vi "main.vi"() -> ()   [LabVIEW 2021]
uses:
  TypeDef/InitCluster.ctl
  <vilib>/express/express shared/transition.llb/Dynamic To Waveform Array.vi
  <vilib>/express/express signal manip/GetorSetDDTAttributes/Set DDT Attributes/SetT0.vi
  <vilib>/express/express signal manip/GetorSetDDTAttributes/Set DDT Attributes/sub Set StartTimeStamp.vi
  <vilib>/express/express shared/transition.llb/Waveform Array To Dynamic.vi
  GlobalVar/GlobalRes.vi
  <vilib>/express/express signal manip/GetorSetDDTAttributes/Set DDT Attributes/Set DDT Properties.xnode
  <vilib>/express/express signal manip/GetorSetDDTAttributes/Set DDT Attributes/Set DDT Attributes.lvlib
panel:
  out "BufPulse":dbl
  out "Number of samples":i32
  out "Rate":dbl
  out "Ilość impulsów":dbl
  out "Czas impulsu":dbl
  out "Info":string
  in  "Stop Button":bool
  in  "Start Button":bool
  in  "Exit Button":bool
  in  "Tab Control":T1(tab)
  in  "Chart/Graph":bool
  in  "Ilosc_ai":u8=1 min=1 max=5
  in  "Offset":dbl=2.0 min=-2.0 max=2.0 step=0.1
  in  "Frequency":dbl=10.1
  in  "Amplitude":dbl=0.2 min=-0.2 max=0.2
  in  "Phase":dbl
  in  "Radio Buttons":T2(radio)
  in  "Test sygnału":bool
  in  "Offset SinZak":dbl=4.0 caption="Offset"
  in  "Funk_pom":enum32{"F:1", "F:2"}(radio)
  in  "fclkknob":dbl(knob) scale=0.0..3.0
  in  "fclk-zad":dbl=35.0 min=35.0 max=600.0
  in  "Uref":dbl=0.5 min=0.5 max=1.0
  out "SygZad Podg":dynamicdata(graph)
  in  "Num of samp":i32=1000
  in  "rate [Hz]":dbl=2000.0
  in  "rate [Hz] 2":dbl=2000.0
  in  "Num of samp 2":i32=1000
  out "T1+T2":dbl
  out "CE 2":dbl(graph)
  out "IN HI / IN LO":dynamicdata(graph)
  out "INT IN":dynamicdata(graph)
  out "INT OUT":dynamicdata(graph)
  out "GATE":dynamicdata(graph)
  out "COUNTER":dynamicdata(graph)
  out "IN HI/ IN LO":dynamicdata(graph)
  out "GATE":dynamicdata(graph)
  out "INT OUT":dynamicdata(graph)
  out "INT IN":dynamicdata(graph)
  out "COUNTER":dbl[](graph)
  # "Duration of\nopen gate"
  # "Number of impulses\nduring open gate"
  # "Rate and number of samples of \neach analog input channel"
  # "Double integration A/D converter test software"
  # "Institute of Automation - Department of Measurements and Control Systems"
  # "Step 1. Configure the input signal"
  # "In Alternating signal \"Offset\" means a peaks of sine wave.\nFor example, if \"Offset\" is set to 2,\nthen wave will be oscillate between -2 and 2.\nIn Noise signal, \"Offset means a value  \naround which the amplitude value oscillates."
  # "Test the signal"
  # "Step 2. Enter parameters of frequency and operating mode"
  # "Chose Chart\nor Graph"
  # "Number of\nanalog inputs"
  # "Noise signal"
  # "Constant signal"
  # "Alternating signal"
  # "Measurement\nfunctions of A/D"
  # "Frequency of\nA/D clock"
  # "If the pulse frequency is set to EXT\nor 35-600kHz, enter the set value in kHz here"
  # "Reference\nVoltage"
  # "Input signal preview"
  # "Number of Pulses per cycle"
  # "Real signal entering the converter"
  # "Integrator input"
  # "Integrator Output"
  # "Gate"
  # "Pulses"
  # "Integrator input"
  # "Integrator Output"
  # "Gate"
  # "Pulses"
  # "Real signal entering the converter"
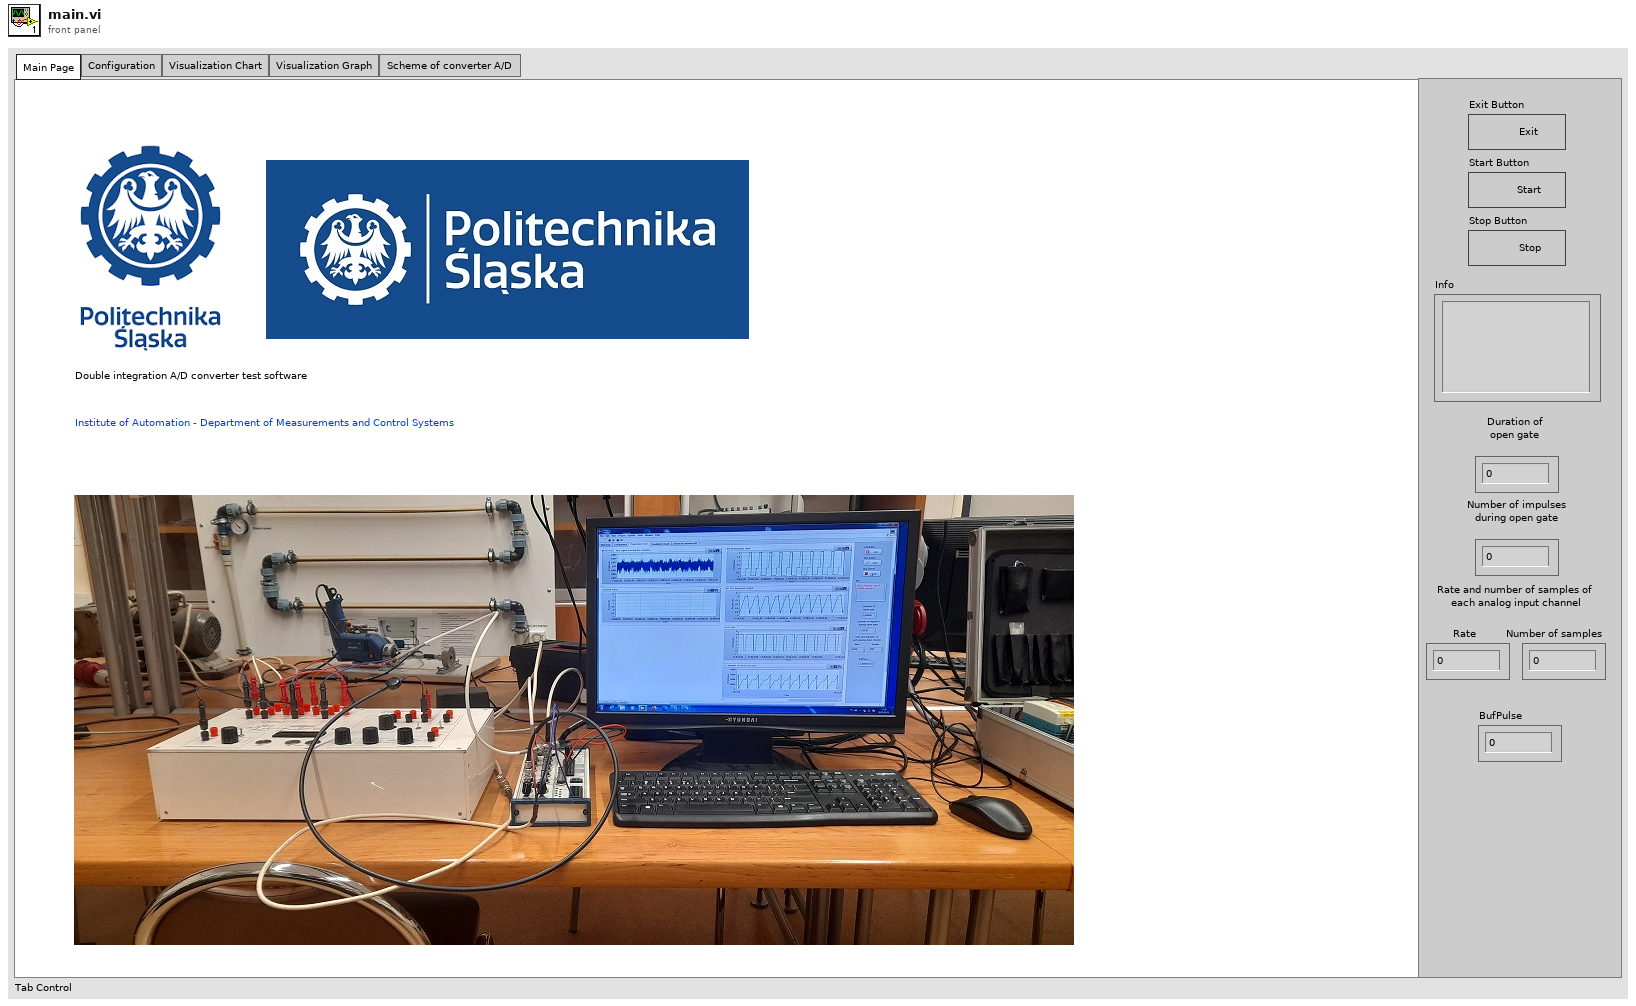
[diagram p1: front panel]
types:
  T1 = enum32{"Main Page", "Configuration", "Visualization Chart", "Visualization Graph", "Scheme of converter A/D "}
  T2 = enum32{"Sygnał przemienny", "Sygnał stały", "Sygnał zakłócony"}
  T3 = enum32{"Invalid", "Standard", "Closed", "Hidden", "Minimized", "Maximized"}
  T4 = enum32{"invalid app kind", "Development System", "Run Time System", "Student Edition", "Embedded LabVIEW", "Evaluation", "Custom"}
  T5 = enum8{"Enabled", "Disabled", "Disabled and Grayed Out"}
  T6 = typedef "InitCluster.ctl" = cluster{"Offset Ref":refnum<vi>, "Frequency Ref":refnum<vi>, "Amplitude Ref":refnum<vi>, "Phase Ref":refnum<vi>, "SygZad Podg Ref":refnum<vi>, "Test sygnału Ref":refnum<vi>, "Radio Buttons Ref":refnum<vi>, "Offset sin zakłócającej Ref":refnum<vi>, "fclkknob Ref":refnum<vi>, "fclk-zad Ref":refnum<vi>, "Info Ref":refnum<vi>}
  T7 = cluster{"Core":cluster{"Current VI Reference":refnum<vi>, "Close Panel on Exit?":bool}, "ClusterOUT":T6}
  T8 = cluster{"Current VI Reference":refnum<vi>, "Close Panel on Exit?":bool}
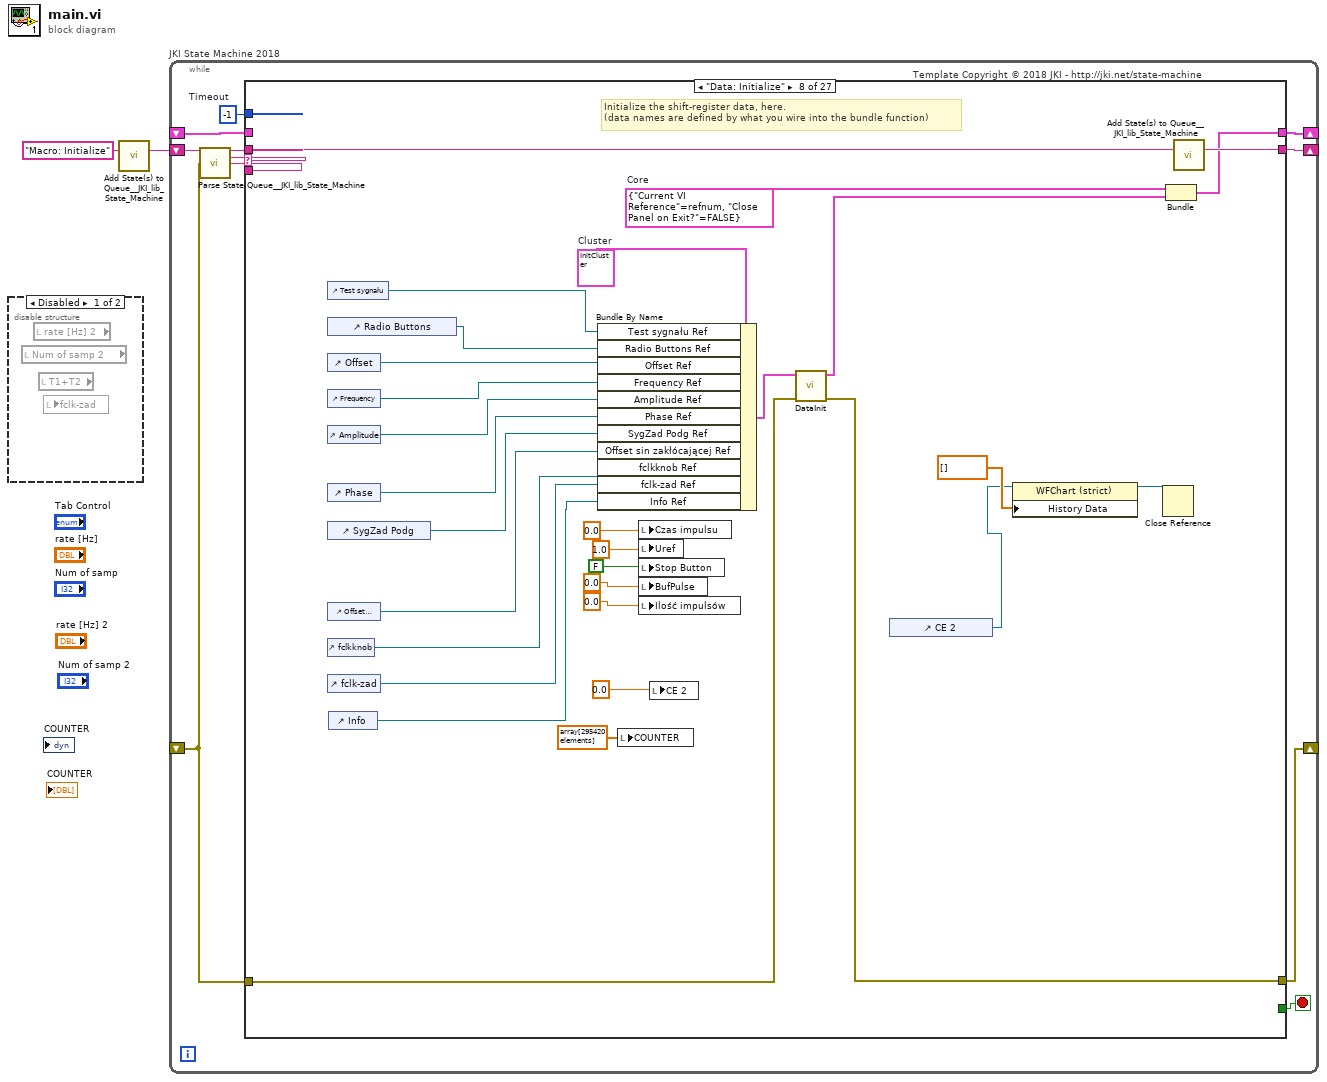
[diagram p0: block diagram]
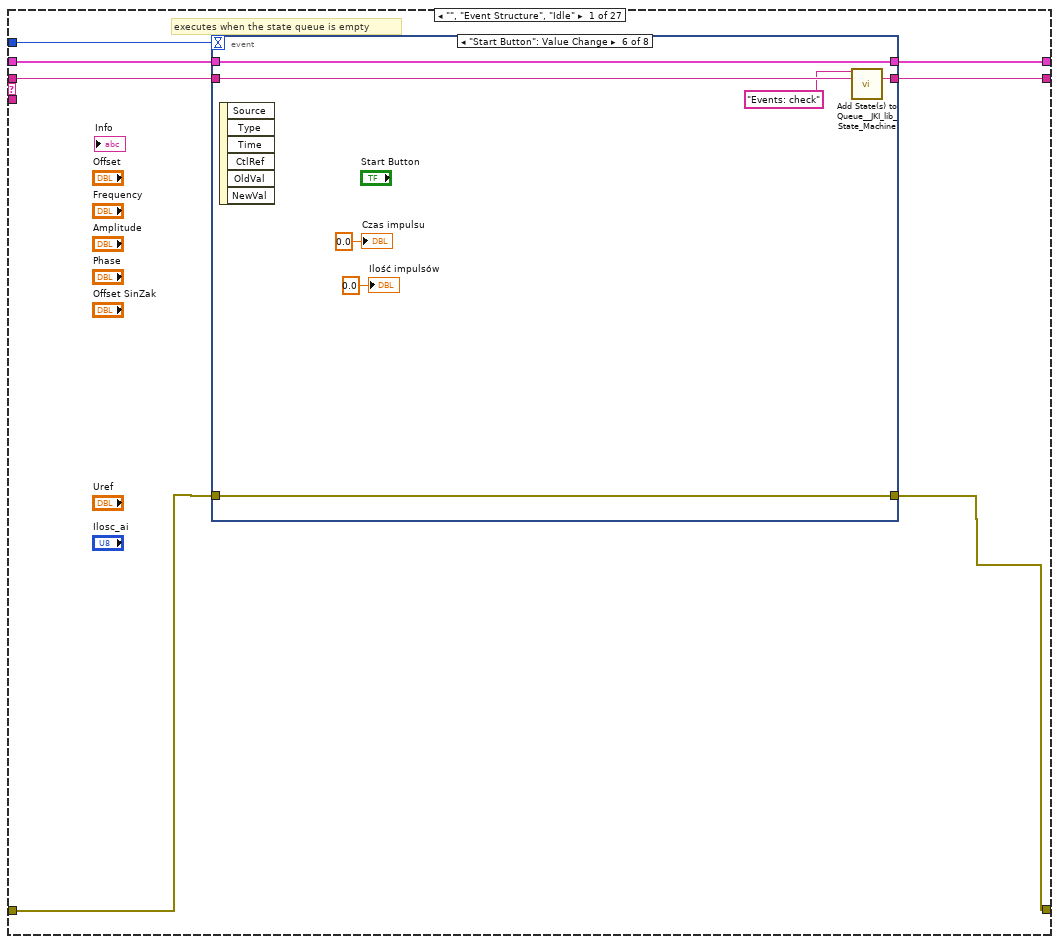
[diagram p3: hidden frame]
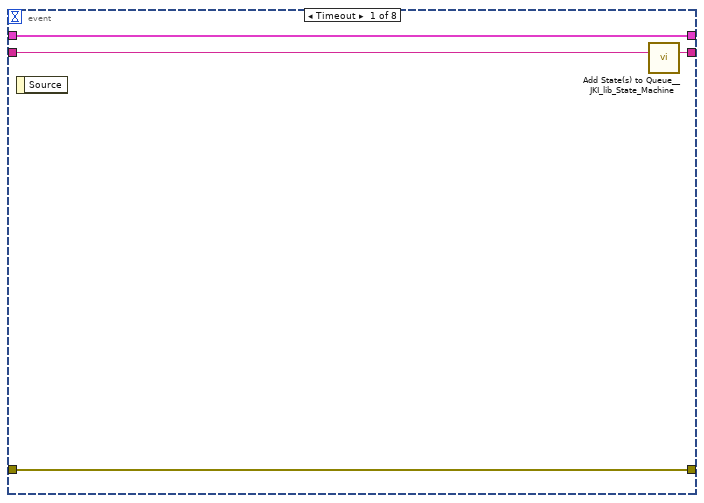
[diagram p4: hidden frame]
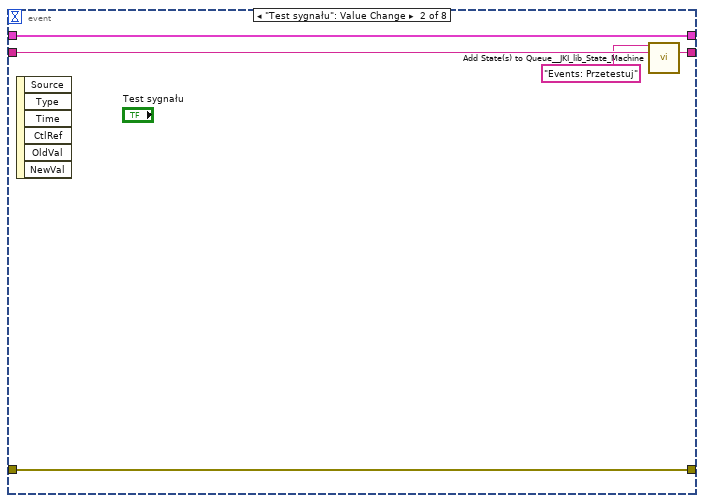
[diagram p5: hidden frame]
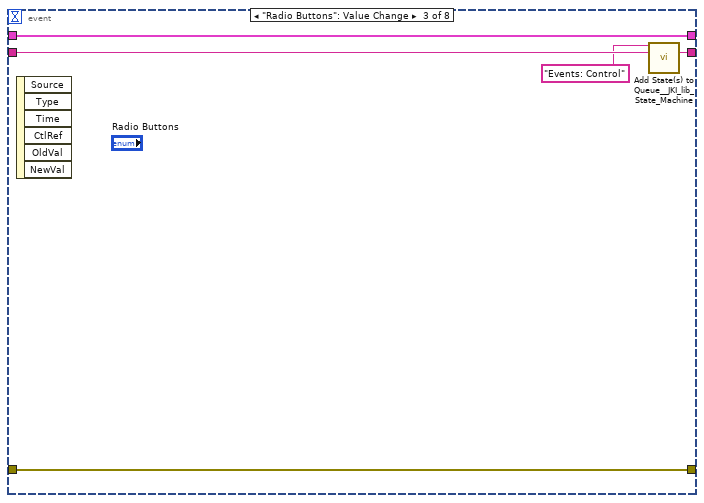
[diagram p6: hidden frame]
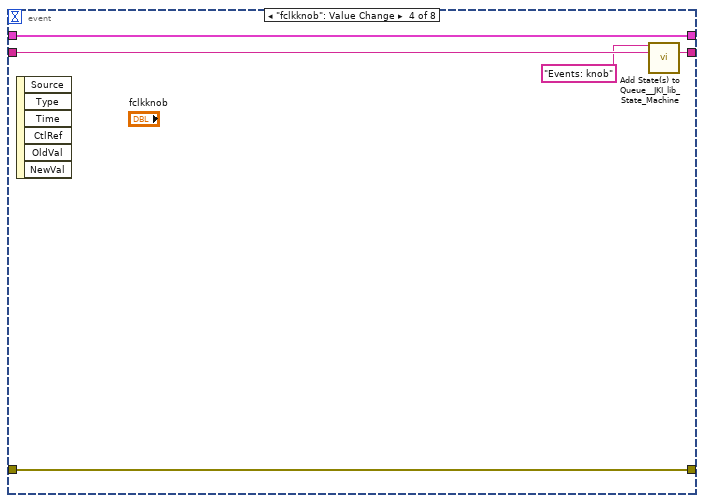
[diagram p7: hidden frame]
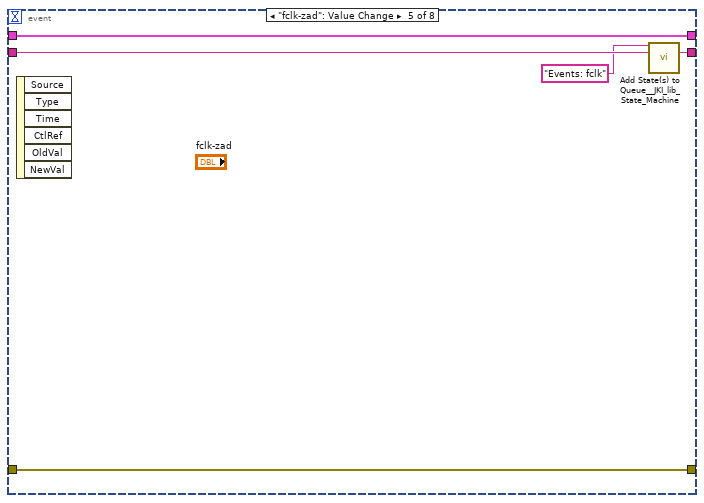
[diagram p8: hidden frame]
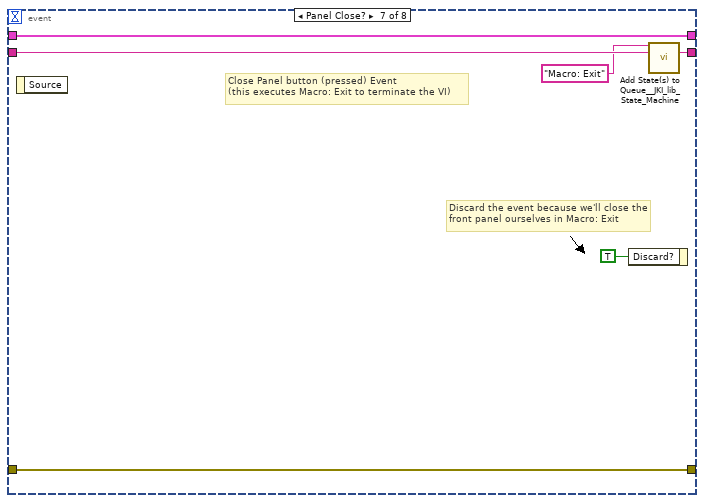
[diagram p9: hidden frame]
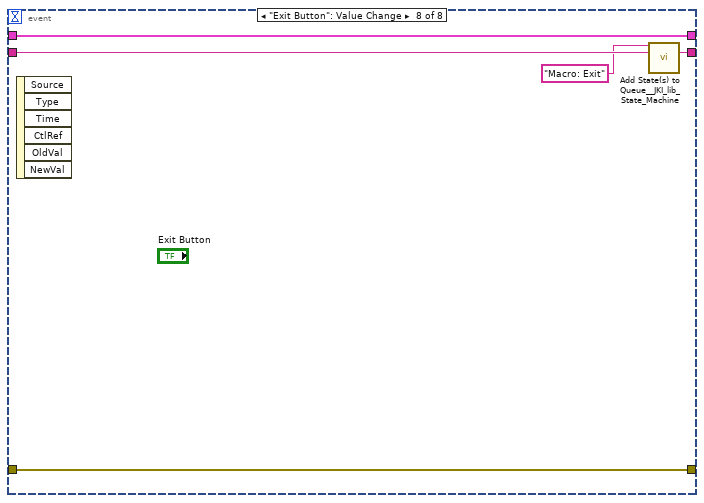
[diagram p10: hidden frame]
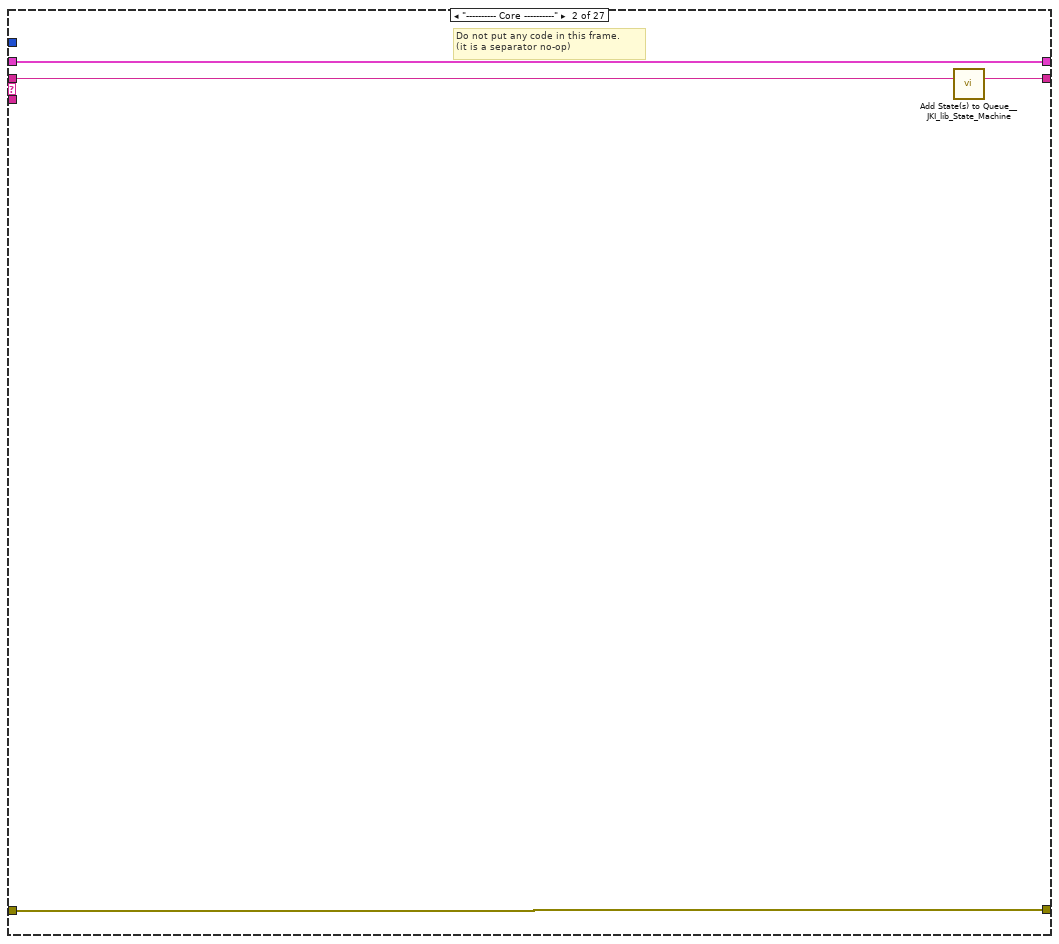
[diagram p11: hidden frame]
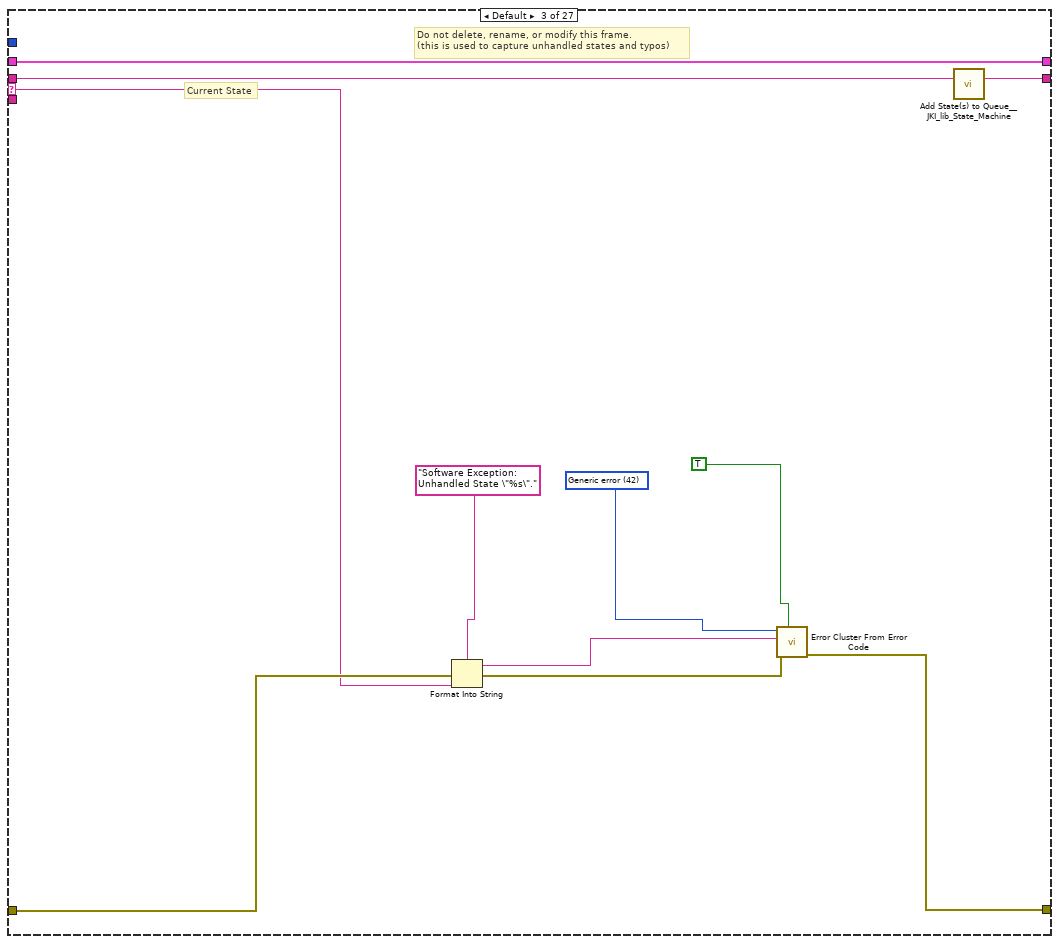
[diagram p12: hidden frame]
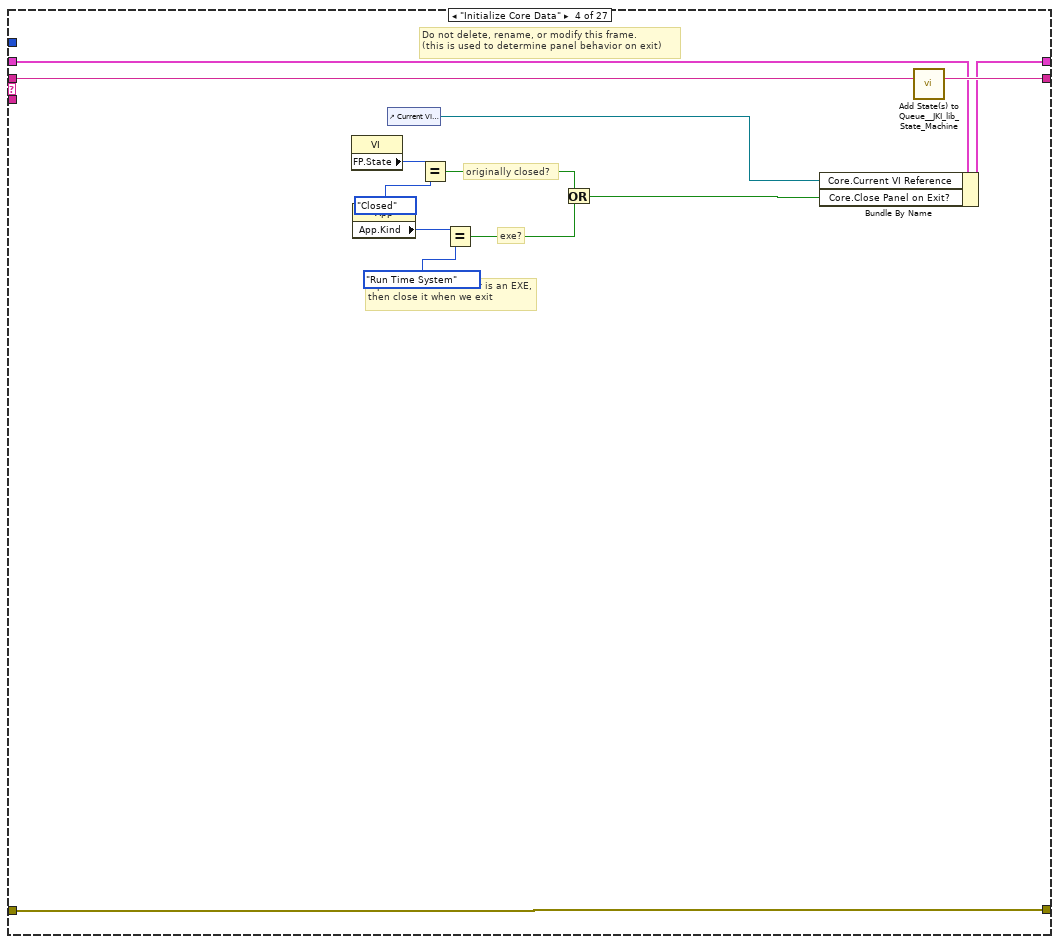
[diagram p13: hidden frame]
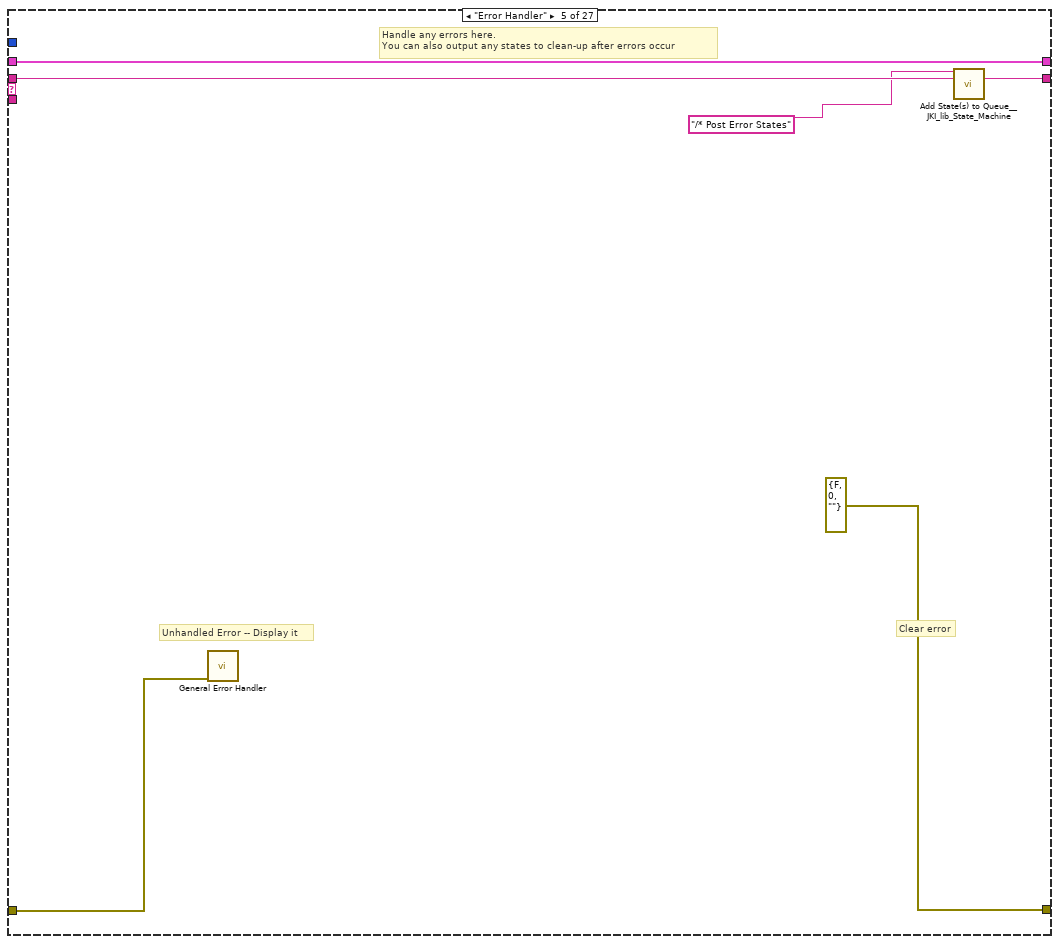
[diagram p14: hidden frame]
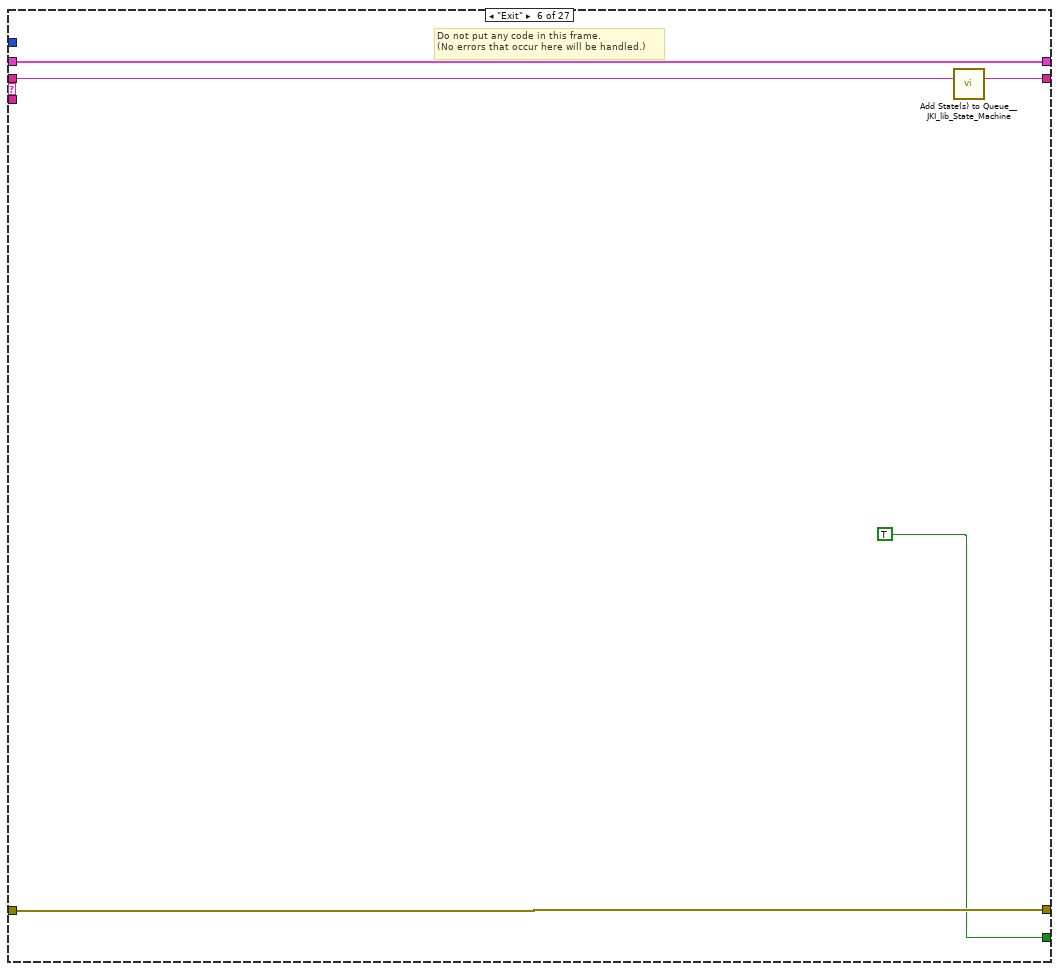
[diagram p15: hidden frame]
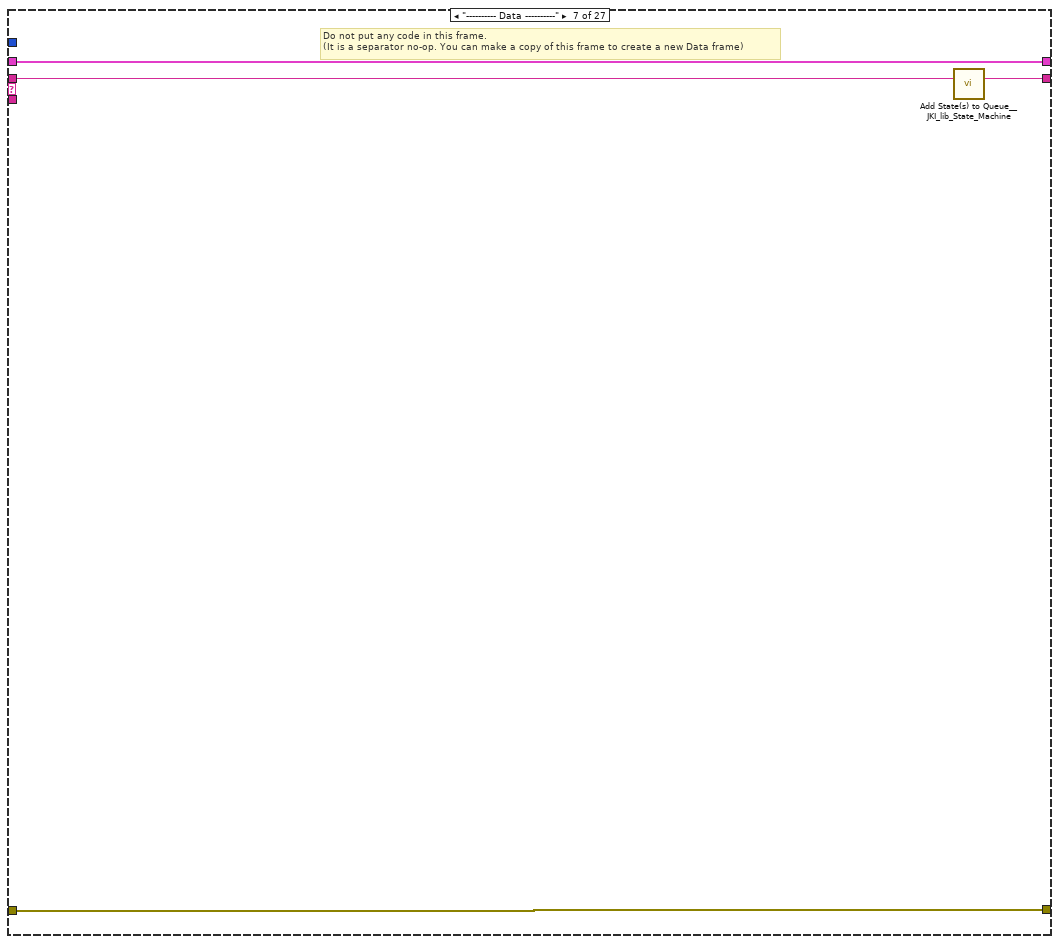
[diagram p16: hidden frame]
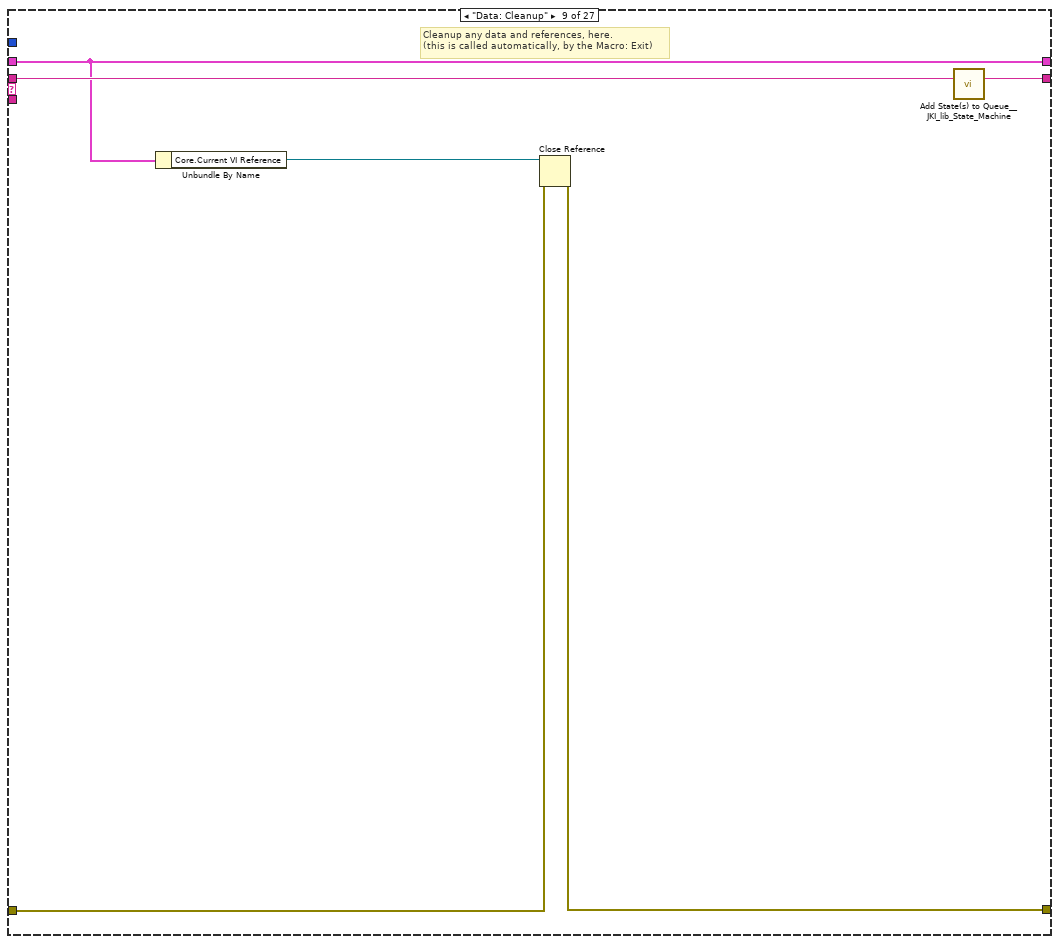
[diagram p17: hidden frame]
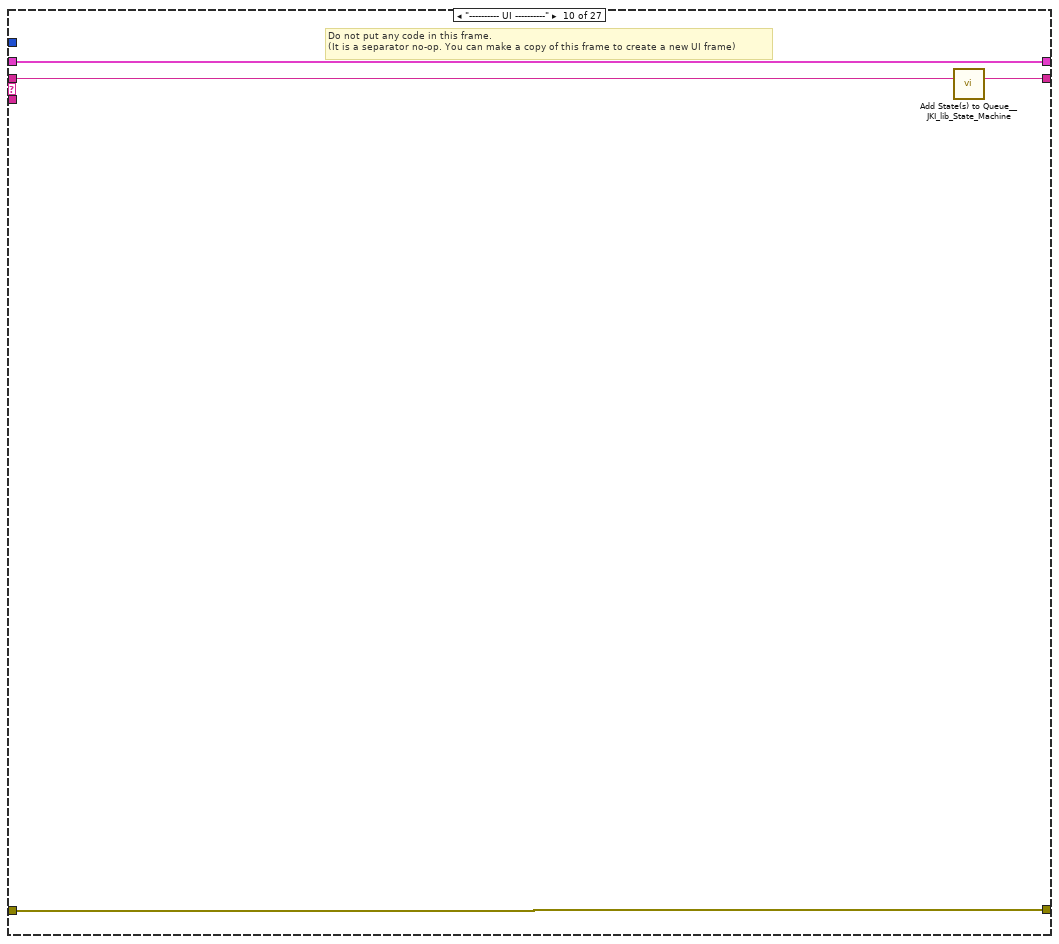
[diagram p18: hidden frame]
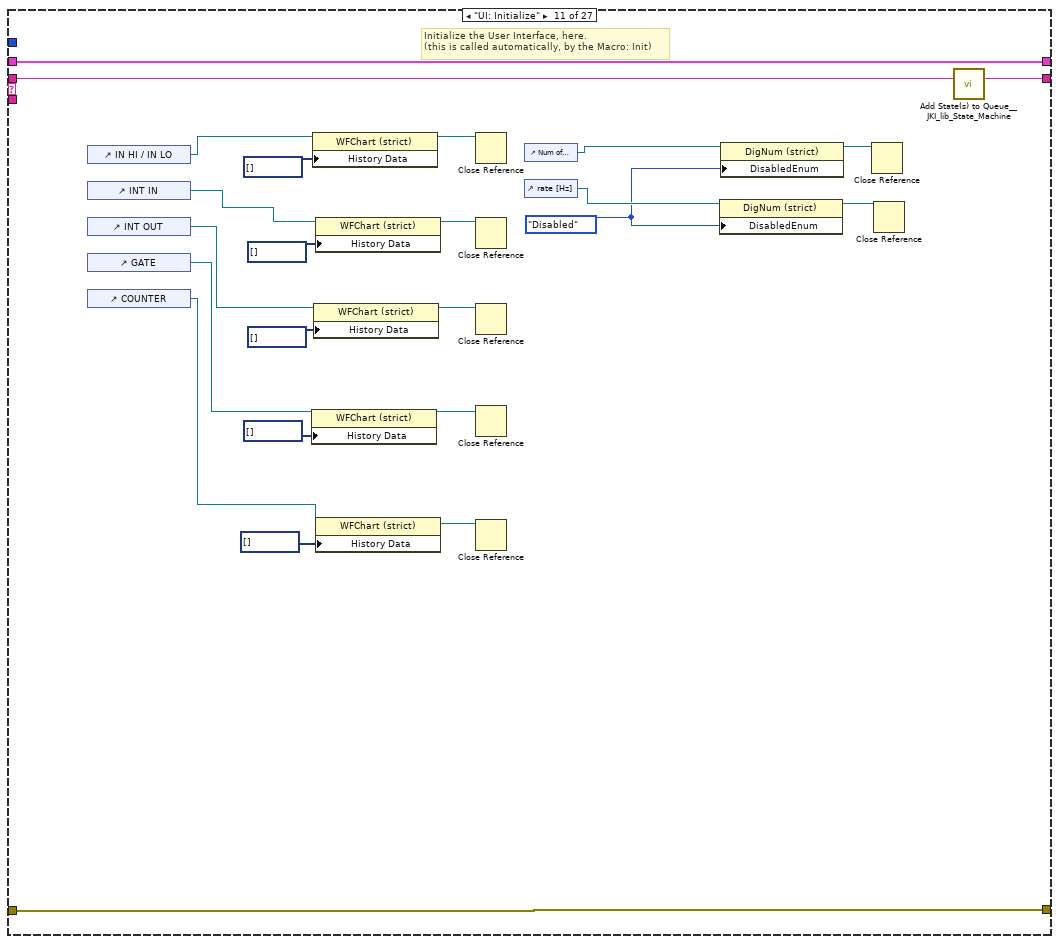
[diagram p19: hidden frame]
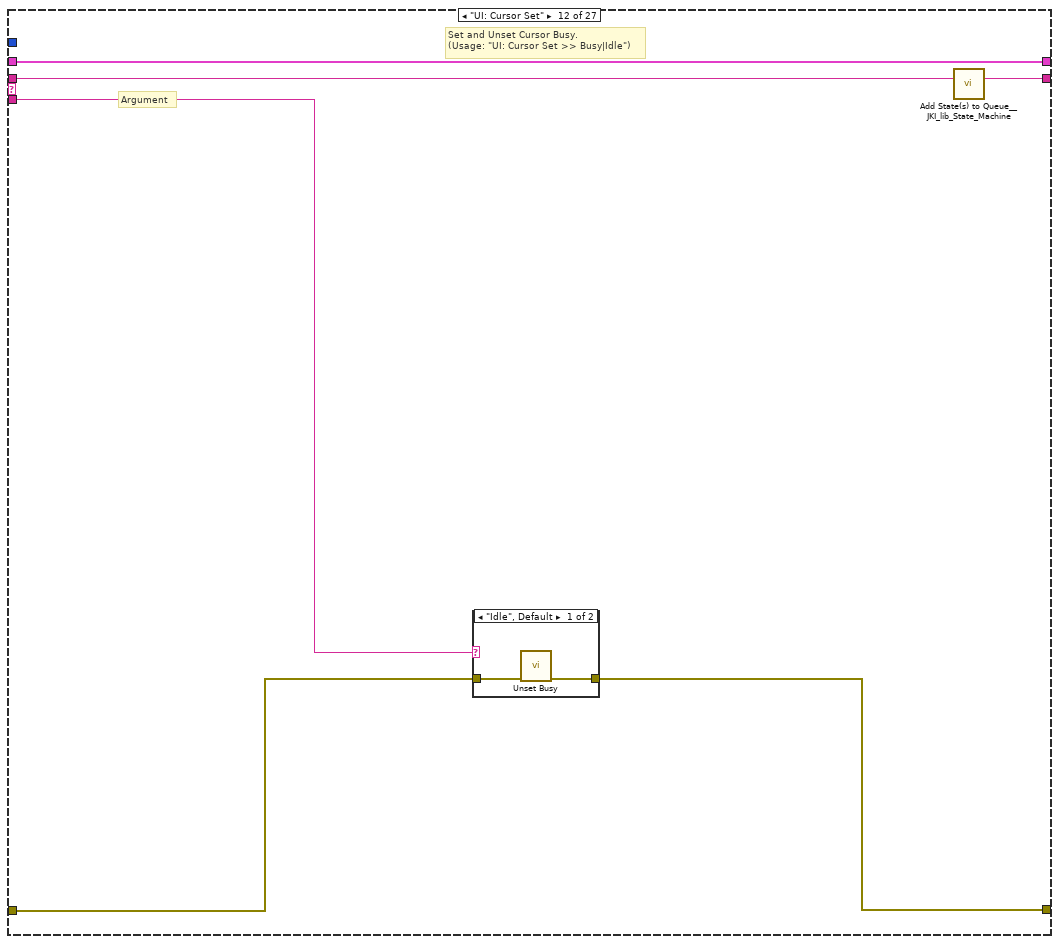
[diagram p20: hidden frame]
diagram:
  n1 = disable-structure shown="Disabled" {
    frame Disabled {
      n2 = local read "Num of samp 2"() -> ()  [unwired: 1 out]
      n3 = local read "rate [Hz] 2"() -> ()  [unwired: 1 out]
      n4 = local read "T1+T2"() -> ()  [unwired: 1 out]
      n5 = local read "fclk-zad"() -> ()  [unwired: 1 in]
    }
    frame Enabled {
    }
  }
  n6 = call <vilib>:"Add State(s) to Queue__JKI_lib_State_Machine.vi"("State(s) in (\"\")"="Macro: Initialize") -> ("States Out"=w2:string)  [unwired: 14 in]
  n7 = while "JKI State Machine 2018" {
    shift-right: [w7] -> _
    shift-left: _ -> [w6]
    shift-right: [w9] -> _
    shift-left: _ -> [w4]
    shift-right: [w8] -> _
    shift-left: w2 -> [w10]
    stop <- w3 stop-if-true
    w5 = -1  # Timeout
    # "Template Copyright © 2018 JKI - http://jki.net/state-machine"
    n8 = call <vilib>:"Parse State Queue__JKI_lib_State_Machine.vi"("State Queue"=w10, "Error In (no error)"=w4) -> ("Remaining States"=w12:string, "Current State"=w13:string, "Arguments"=w11:string)  [unwired: 11 in]
    n9 = case shown="\"Data: Initialize\"" w13 {
      selector: w13 -> [_ _ w67 _ _ _ _ _ _ _ _ _ _ _ _ _ _ _ _ _ _ _ _ _ _ _ _]
      tunnel: w12 -> [w20 w66 w71 w90 w96 w101 w105 w135 w141 w145 w169 w175 w186 w255 w260 w270 w274 w285 w337 w401 w441 w452 w551 w575 w639 w670 w700]
      tunnel: w11 -> [_ _ _ _ _ _ _ _ _ _ _ w170 w180 _ _ _ _ _ _ _ _ _ _ _ _ _ _]
      tunnel: w6 -> [w18 w63 w69 w83 w93 w99 w102 _ w136 w142 w167 w173 w182 w252 w257 w267 w271 w280 w334 w398 w439 w450 w549 w573 w636 w667 w698]
      tunnel: [w17 w64 w73 w87 errorcluster {"status"=FALSE, "code"=0, "source"=""} ("error out") w98 w103 w125 w137 w143 w166 w171 w183 w253 w258 w268 w272 w282 w332 w390 w436 w443 w518 w572 w624 w655 w686] -> w9
      tunnel: w4 -> [w16 w64 w72 w87 w92 w98 w103 w126 w138 w143 w166 w172 w184 w253 w258 w268 w272 w277 w333 w396 w438 w444 w546 w572 w624 w655 w685]
      tunnel: [w19 w65 w70 w89 w95 w100 w104 w134 w140 w144 w168 w174 w185 w254 w259 w269 w273 w284 w336 w400 w440 w451 w550 w574 w638 w669 w699] -> w8
      tunnel: [_ _ _ _ _ TRUE _ _ _ _ _ _ _ _ _ _ _ _ _ _ _ _ _ _ _ _ _] -> w3
      tunnel: [w15 w63 w69 w88 w93 w99 w102 w133 w136 w142 w167 w173 w182 w252 w257 w267 w271 w280 w334 w398 w439 w450 w549 w573 w636 w667 w698] -> w7
      tunnel: w5 -> [w14 _ _ _ _ _ _ _ _ _ _ _ _ _ _ _ _ _ _ _ _ _ _ _ _ _ _]
      frame "", "Event Structure", "Idle" {
        # "executes when the state queue is empty"
        n10 = event shown="[5] \"Start Button\": Value Change" {
          selector: _ -> [_ _ _ _ _ _ _ _]
          dyn-events: _ -> [_ _ _ _ _ _ _ _]
          timeout: w14 -> [_ _ _ _ _ _ _ _]
          tunnel: w20 -> [w24 w29 w34 w39 w44 w51 w57 w62]
          tunnel: [w23 w28 w33 w38 w43 w50 w56 w61] -> w19
          tunnel: w18 -> [w21 w26 w31 w36 w41 w48 w54 w59]
          tunnel: [w22 w27 w32 w37 w42 w49 w55 w60] -> w17
          tunnel: w16 -> [w22 w27 w32 w37 w42 w49 w55 w60]
          tunnel: [w21 w26 w31 w36 w41 w48 w54 w59] -> w15
          event Timeout {
            n11 = event-data() -> ()  [unwired: 1 in, 1 out]
            n12 = call <vilib>:"Add State(s) to Queue__JKI_lib_State_Machine.vi"("State(s) in (\"\")"=w24) -> ("States Out"=w23:string)  [unwired: 14 in]
          }
          event "Test sygnału": Value Change {
            n13 = event-data() -> ()  [unwired: 1 in, 6 out]
            n14 = call <vilib>:"Add State(s) to Queue__JKI_lib_State_Machine.vi"("State(s) in Front (\"\")"="Events: Przetestuj", "State(s) in (\"\")"=w29) -> ("States Out"=w28:string)  [unwired: 13 in]
          }
          event "Radio Buttons": Value Change {
            n15 = event-data() -> ()  [unwired: 1 in, 6 out]
            n16 = call <vilib>:"Add State(s) to Queue__JKI_lib_State_Machine.vi"("State(s) in Front (\"\")"="Events: Control", "State(s) in (\"\")"=w34) -> ("States Out"=w33:string)  [unwired: 13 in]
          }
          event "fclkknob": Value Change {
            n17 = event-data() -> ()  [unwired: 1 in, 6 out]
            n18 = call <vilib>:"Add State(s) to Queue__JKI_lib_State_Machine.vi"("State(s) in Front (\"\")"="Events: knob", "State(s) in (\"\")"=w39) -> ("States Out"=w38:string)  [unwired: 13 in]
          }
          event "fclk-zad": Value Change {
            n19 = event-data() -> ()  [unwired: 1 in, 6 out]
            n20 = call <vilib>:"Add State(s) to Queue__JKI_lib_State_Machine.vi"("State(s) in Front (\"\")"="Events: fclk", "State(s) in (\"\")"=w44) -> ("States Out"=w43:string)  [unwired: 13 in]
          }
          event "Start Button": Value Change {
            n21 = event-data() -> ()  [unwired: 1 in, 6 out]
            n22 = call <vilib>:"Add State(s) to Queue__JKI_lib_State_Machine.vi"("State(s) in Front (\"\")"="Events: check", "State(s) in (\"\")"=w51) -> ("States Out"=w50:string)  [unwired: 13 in]
            "Czas impulsu" <- 0.0 ("Czas impulsu")
            "Ilość impulsów" <- 0.0 ("Ilość impulsów")
          }
          event Panel Close? {
            # "Discard the event because we'll close the front panel ourselves in Macro: Exit"
            # "Close Panel button (pressed) Event\n(this executes Macro: Exit to terminate the VI)"
            n23 = event-data() -> ()  [unwired: 1 in, 1 out]
            n24 = event-data("Discard?"=TRUE) -> ()  [unwired: 1 in, 1 out]
            n25 = call <vilib>:"Add State(s) to Queue__JKI_lib_State_Machine.vi"("State(s) in Front (\"\")"="Macro: Exit", "State(s) in (\"\")"=w57) -> ("States Out"=w56:string)  [unwired: 13 in]
          }
          event "Exit Button": Value Change {
            n26 = event-data() -> ()  [unwired: 1 in, 6 out]
            n27 = call <vilib>:"Add State(s) to Queue__JKI_lib_State_Machine.vi"("State(s) in Front (\"\")"="Macro: Exit", "State(s) in (\"\")"=w62) -> ("States Out"=w61:string)  [unwired: 13 in]
          }
        }
      }
      frame "---------- Core ----------" {
        # "Do not put any code in this frame.\n(it is a separator no-op)"
        n28 = call <vilib>:"Add State(s) to Queue__JKI_lib_State_Machine.vi"("State(s) in (\"\")"=w66) -> ("States Out"=w65:string)  [unwired: 14 in]
      }
      frame Default {
        w76 = 42 items=["No error", "Argument error", "Memory is full", "Out of zone", "End of file", "File already open", "Generic file I/O error", "File not found", "File permission error", "Disk is full", "Duplicate path", "Too many files open", "System feature not enabled", "Resource file not found", "Cannot add resource", "Resource not found", "Image not found", "Image memory error", "Pen does not exist", "Config type invalid", "Config token not found", "Config parse error", "Config memory error", "Bad external code format", "Bad external code offset", "External code not present", "Null window", "Destroy window error", "Null menu", "Print aborted", "Bad print record", "Print driver error", "Windows error during printing", "Memory error during printing", "Print dialog error", "Generic print error", "Invalid device refnum", "Device not found", "Device parameter error", "Device unit error", "Cannot open device", "Device call aborted", "Generic error", "Cancelled by user", "Object ID too low", "Object ID too high", "Object not in heap", "Unknown heap", "Unknown object (invalid DefProc)", "Unknown object (DefProc not in table)", "Message out of range", "Invalid (null) method", "Unknown message", "Manager call not supported", "Bad address", "Network operation in progress", "Network operation timed out", "Connection is busy", "Network attribute not supported", "Network error", "Address in use", "System out of memory", "Connection aborted", "Connection refused", "Not connected", "Already connected", "Connection closed", "Initialization error (interapplication manager)", "Bad occurrence", "Wait on unbound occurrence handler", "Occurrence queue overflow", "Datalog type conflict", "Unused", "Unrecognized type (interapplication manager)", "Memory corrupt", "Failed to make temporary DLL", "Old CIN version", "Drag socket not found", "Failed to load drop-object", "Failed to register OLE object", "Failed to release OLE object", "Format specifier type mismatch", "Unknown format specifier", "Too few format specifiers", "Too many format specifiers", "Scan failed", "Newer CIN version", "Error converting to variant", "Runtime menu error", "Password tampered", "Variant attribute not found", "Incompatible variant data type", "Event data is not available", "Event Store is not present", "Occurrence is not found", "Event Queue is not created", "Event info is not available", "Refnum passed is NULL", "Error retrieving Class GUID", "Error retrieving CoClass GUID", "Error retrieving TypeLib GUID.", "Bad built application magic bytes.", "Specific driver is different from the specific driver associated with the Logical Name.", "There is no session opened to the class driver.", "Max Error", "MAX - Error with config objects", "MAX - Error loading configuration", "MAX - Group not supported"]
        # "Current State"
        # "Do not delete, rename, or modify this frame.\n(this is used to capture unhandled states and typos)"
        n29 = Format Into String(format string="Software Exception: Unhandled State \"%s\"." ("message"), error in=w72, w67) -> (resulting string=w75:string, error out=w74:errorcluster)  [unwired: 1 in]
        n30 = call <vilib>:"Error Cluster From Error Code.vi"("show call chain? (False)"=TRUE, "error in (no error)"=w74, "error message (\"\")"=w75, "error code (0)"=w76) -> ("error out"=w73:errorcluster)  [unwired: 5 in]
        n31 = call <vilib>:"Add State(s) to Queue__JKI_lib_State_Machine.vi"("State(s) in (\"\")"=w71) -> ("States Out"=w70:string)  [unwired: 14 in]
      }
      frame "Initialize Core Data" {
        # "Do not delete, rename, or modify this frame.\n(this is used to determine panel behavior on exit)"
        # "originally closed?"
        # "exe?"
        # "If panel starts closed or is an EXE, then close it when we exit"
        n32 = property class="VI"() -> ("FP.State"=w80:T3)  [unwired: 2 in, 2 out]
        n33 = property class="App"() -> ("App.Kind"=w86:T4)  [unwired: 2 in, 2 out]
        n34 = control-ref of="Current VI Reference"() -> (w81:refnum<vi>)
        n35 = Equal?(x=w80, y=T3."Closed" ("Front Panel Window:State")) -> (x = y?=w78:bool)
        n36 = Equal?(x=w86, y=T4."Run Time System" ("Application:Kind")) -> (x = y?=w84:bool)
        n37 = Or(x=w78, y=w84) -> (x .or. y?=w82:bool)
        n38 = Bundle By Name(cluster=w83, "Core.Current VI Reference"=w81, "Core.Close Panel on Exit?"=w82) -> (w88:T7)
        n39 = call <vilib>:"Add State(s) to Queue__JKI_lib_State_Machine.vi"("State(s) in (\"\")"=w90) -> ("States Out"=w89:string)  [unwired: 14 in]
      }
      frame "Error Handler" {
        # "Unhandled Error -- Display it"
        # "Handle any errors here.\nYou can also output any states to clean-up after errors occur"
        # "Clear error"
        n40 = call <vilib>:"General Error Handler.vi"("error in (no error)"=w92) -> ()  [unwired: 10 in, 5 out]
        n41 = call <vilib>:"Add State(s) to Queue__JKI_lib_State_Machine.vi"("State(s) in Front (\"\")"="/* Post Error States", "State(s) in (\"\")"=w96) -> ("States Out"=w95:string)  [unwired: 13 in]
      }
      frame "Exit" {
        # "Do not put any code in this frame.\n(No errors that occur here will be handled.)"
        n42 = call <vilib>:"Add State(s) to Queue__JKI_lib_State_Machine.vi"("State(s) in (\"\")"=w101) -> ("States Out"=w100:string)  [unwired: 14 in]
      }
      frame "---------- Data ----------" {
        # "Do not put any code in this frame.\n(It is a separator no-op. You can make a copy of this frame to create a new Data frame)"
        n43 = call <vilib>:"Add State(s) to Queue__JKI_lib_State_Machine.vi"("State(s) in (\"\")"=w105) -> ("States Out"=w104:string)  [unwired: 14 in]
      }
      frame "Data: Initialize" {
        w131 = T6 {"Offset Ref"=refnum, "Frequency Ref"=refnum, "Amplitude Ref"=refnum, "Phase Ref"=refnum, "SygZad Podg Ref"=refnum, "Test sygnału Ref"=refnum, "Radio Buttons Ref"=refnum, "Offset sin zakłócającej Ref"=refnum, "fclkknob Ref"=refnum, "fclk-zad Ref"=refnum, "Info Ref"=refnum}  # Cluster
        w132 = T8 {"Current VI Reference"=refnum, "Close Panel on Exit?"=FALSE}  # Core
        # "Initialize the shift-register data, here.\n(data names are defined by what you wire into the bundle function)"
        n44 = control-ref of="Test sygnału"() -> (w121:refnum<vi>)
        n45 = control-ref of="Radio Buttons"() -> (w120:refnum<vi>)
        n46 = control-ref of="Offset"() -> (w130:refnum<vi>)
        n47 = control-ref of="Frequency"() -> (w129:refnum<vi>)
        n48 = control-ref of="Amplitude"() -> (w128:refnum<vi>)
        n49 = control-ref of="Phase"() -> (w127:refnum<vi>)
        n50 = control-ref of="SygZad Podg"() -> (w122:refnum<vi>)
        n51 = control-ref of="Offset SinZak"() -> (w119:refnum<vi>)
        n52 = control-ref of="fclkknob"() -> (w118:refnum<vi>)
        n53 = control-ref of="fclk-zad"() -> (w117:refnum<vi>)
        n54 = control-ref of="Info"() -> (w116:refnum<vi>)
        n55 = Bundle By Name(cluster=w131, "Test sygnału Ref"=w121, "Radio Buttons Ref"=w120, "Offset Ref"=w130, "Frequency Ref"=w129, "Amplitude Ref"=w128, "Phase Ref"=w127, "SygZad Podg Ref"=w122, "Offset sin zakłócającej Ref"=w119, "fclkknob Ref"=w118, "fclk-zad Ref"=w117, "Info Ref"=w116) -> (w124:T6)
        n56 = local write "COUNTER"(dbl[] array[295420 elements] ("COUNTER")) -> ()
        n57 = local write "Czas impulsu"(0.0 ("Czas impulsu")) -> ()
        n58 = local write "Uref"(1.0 ("Uref")) -> ()
        n59 = local write "Stop Button"(FALSE ("Stop Button")) -> ()
        n60 = local write "BufPulse"(0.0 ("Numeric")) -> ()
        n61 = local write "Ilość impulsów"(0.0 ("Ilość impulsów")) -> ()
        n62 = local write "CE 2"(0.0 ("CE2")) -> ()
        n63 = call "DataInit.vi"("error in (no error)"=w126, "ClusterIN"=w124) -> ("error out"=w125:errorcluster, "ClusterOUT"=w123:T6)  [unwired: 8 in]
        n64 = control-ref of="CE 2"() -> (w107:refnum<vi>)
        n65 = property class="WFChart (strict)"(reference=w107, "History Data"=dbl[] []) -> (reference out=w110:refnum<vi>)  [unwired: 1 in, 1 out]
        n66 = Close Reference(reference=w110) -> ()  [unwired: 1 in, 1 out]
        n67 = Bundle("Core"=w132, "ClusterOUT"=w123) -> (w133:T7)  [unwired: 1 in]
        n68 = call <vilib>:"Add State(s) to Queue__JKI_lib_State_Machine.vi"("State(s) in (\"\")"=w135) -> ("States Out"=w134:string)  [unwired: 14 in]
      }
      frame "Data: Cleanup" {
        # "Cleanup any data and references, here.\n(this is called automatically, by the Macro: Exit)"
        n69 = Unbundle By Name(w136) -> ("Core.Current VI Reference"=w139:refnum<vi>)
        n70 = Close Reference(reference=w139, error in (no error)=w138) -> (error out=w137:errorcluster)
        n71 = call <vilib>:"Add State(s) to Queue__JKI_lib_State_Machine.vi"("State(s) in (\"\")"=w141) -> ("States Out"=w140:string)  [unwired: 14 in]
      }
      frame "---------- UI ----------" {
        # "Do not put any code in this frame.\n(It is a separator no-op. You can make a copy of this frame to create a new UI frame)"
        n72 = call <vilib>:"Add State(s) to Queue__JKI_lib_State_Machine.vi"("State(s) in (\"\")"=w145) -> ("States Out"=w144:string)  [unwired: 14 in]
      }
      frame "UI: Initialize" {
        w148 = T5."Disabled" ("Disabled")
        # "Initialize the User Interface, here.\n(this is called automatically, by the Macro: Init)"
        n73 = control-ref of="IN HI / IN LO"() -> (w165:refnum<vi>)
        n74 = control-ref of="INT IN"() -> (w163:refnum<vi>)
        n75 = control-ref of="INT OUT"() -> (w159:refnum<vi>)
        n76 = control-ref of="GATE"() -> (w158:refnum<vi>)
        n77 = control-ref of="COUNTER"() -> (w157:refnum<vi>)
        n78 = property class="WFChart (strict)"(reference=w158, "History Data"=dynamicdata[] []) -> (reference out=w152:refnum<vi>)  [unwired: 1 in, 1 out]
        n79 = property class="WFChart (strict)"(reference=w165, "History Data"=dynamicdata[] []) -> (reference out=w155:refnum<vi>)  [unwired: 1 in, 1 out]
        n80 = property class="WFChart (strict)"(reference=w159, "History Data"=dynamicdata[] []) -> (reference out=w153:refnum<vi>)  [unwired: 1 in, 1 out]
        n81 = property class="WFChart (strict)"(reference=w163, "History Data"=dynamicdata[] []) -> (reference out=w154:refnum<vi>)  [unwired: 1 in, 1 out]
        n82 = property class="WFChart (strict)"(reference=w157, "History Data"=dynamicdata[] []) -> (reference out=w151:refnum<vi>)  [unwired: 1 in, 1 out]
        n83 = Close Reference(reference=w155) -> ()  [unwired: 1 in, 1 out]
        n84 = Close Reference(reference=w154) -> ()  [unwired: 1 in, 1 out]
        n85 = Close Reference(reference=w153) -> ()  [unwired: 1 in, 1 out]
        n86 = Close Reference(reference=w152) -> ()  [unwired: 1 in, 1 out]
        n87 = Close Reference(reference=w151) -> ()  [unwired: 1 in, 1 out]
        n88 = control-ref of="Num of samp"() -> (w150:refnum<vi>)
        n89 = control-ref of="rate [Hz]"() -> (w149:refnum<vi>)
        n90 = property class="DigNum (strict)"(reference=w149, "DisabledEnum"=w148) -> (reference out=w146:refnum<vi>)  [unwired: 1 in, 1 out]
        n91 = property class="DigNum (strict)"(reference=w150, "DisabledEnum"=w148) -> (reference out=w147:refnum<vi>)  [unwired: 1 in, 1 out]
        n92 = Close Reference(reference=w147) -> ()  [unwired: 1 in, 1 out]
        n93 = Close Reference(reference=w146) -> ()  [unwired: 1 in, 1 out]
        n94 = call <vilib>:"Add State(s) to Queue__JKI_lib_State_Machine.vi"("State(s) in (\"\")"=w169) -> ("States Out"=w168:string)  [unwired: 14 in]
      }
      frame "UI: Cursor Set" {
        # "Argument"
        # "Set and Unset Cursor Busy.\n(Usage: \"UI: Cursor Set >> Busy|Idle\")"
        n95 = case shown="\"Idle\", Default" w170 {
          tunnel: w172 -> [w177 w179]
          tunnel: [w176 w178] -> w171
          frame "Idle", Default {
            n96 = call <vilib>:"Unset Busy.vi"("error in (no error)"=w177) -> ("error out"=w176:errorcluster)  [unwired: 10 in]
          }
          frame "Busy" {
            n97 = call <vilib>:"Set Busy.vi"("error in (no error)"=w179) -> ("error out"=w178:errorcluster)  [unwired: 9 in, 1 out]
          }
        }
        n98 = call <vilib>:"Add State(s) to Queue__JKI_lib_State_Machine.vi"("State(s) in (\"\")"=w175) -> ("States Out"=w174:string)  [unwired: 14 in]
      }
      frame "UI: Front Panel State" {
        # "Argument"
        # "Set Front Panel Open or Closed\n(Usage: \"UI: Front Panel State >> Open|Close\")"
        n99 = Unbundle By Name(w182) -> ("Core.Current VI Reference"=w181:refnum<vi>)
        n100 = case shown="\"Open\", \"Standard\", Default" w180 {
          tunnel: w184 -> [w192 w207 w218 w231 w244]
          tunnel: [w194 w208 w220 w233 w246] -> w183
          tunnel: w181 -> [w193 w205 w219 w232 w245]
          frame "Open", "Standard", Default {
            w187 = T3."Standard" ("State")
            n101 = property class="VI"(reference=w193, error in=w192) -> (reference out=w190:refnum<vi>, error out=w191:errorcluster, "FP.State"=w189:T3)
            n102 = Not Equal?(x=w189, y=w187) -> (x != y?=w188:bool)
            n103 = case shown="False" w188 {
              tunnel: [w198 w200] -> w194
              tunnel: w191 -> [w197 w200]
              tunnel: w190 -> [w196 _]
              tunnel: w187 -> [w195 _]
              frame True {
                n104 = invoke class="VI" method="FP.Open"(reference=w196, error in=w197, "Activate"=TRUE, "State"=w195) -> (error out=w198:errorcluster)  [unwired: 1 in, 4 out]
              }
              frame False {
              }
            }
          }
          frame "Close", "Closed" {
            n105 = property class="VI"(reference=w205, error in=w207) -> (reference out=w204:refnum<vi>, error out=w206:errorcluster, "FP.State"=w202:T3)
            n106 = Not Equal?(x=w202, y=T3."Closed" ("Front Panel Window:State")) -> (x != y?=w201:bool)
            n107 = case shown="True" w201 {
              tunnel: [w209 w212] -> w208
              tunnel: w206 -> [w209 w211]
              tunnel: w204 -> [_ w210]
              frame False {
              }
              frame True {
                n108 = invoke class="VI" method="FP.Close"(reference=w210, error in=w211) -> (error out=w212:errorcluster)  [unwired: 1 in, 2 out]
              }
            }
          }
          frame "Hidden", "Hide" {
            w213 = T3."Hidden" ("State")
            n109 = property class="VI"(reference=w219, error in=w218) -> (reference out=w216:refnum<vi>, error out=w217:errorcluster, "FP.State"=w215:T3)
            n110 = Not Equal?(x=w215, y=w213) -> (x != y?=w214:bool)
            n111 = case shown="True" w214 {
              tunnel: [w224 w225] -> w220
              tunnel: w217 -> [w223 w225]
              tunnel: w216 -> [w222 _]
              tunnel: w213 -> [w221 _]
              frame True {
                n112 = invoke class="VI" method="FP.Open"(reference=w222, error in=w223, "State"=w221) -> (error out=w224:errorcluster)  [unwired: 2 in, 4 out]
              }
              frame False {
              }
            }
          }
          frame "Minimize", "Minimized" {
            w226 = T3."Minimized" ("State")
            n113 = property class="VI"(reference=w232, error in=w231) -> (reference out=w229:refnum<vi>, error out=w230:errorcluster, "FP.State"=w228:T3)
            n114 = Not Equal?(x=w228, y=w226) -> (x != y?=w227:bool)
            n115 = case shown="True" w227 {
              tunnel: [w237 w238] -> w233
              tunnel: w230 -> [w236 w238]
              tunnel: w229 -> [w235 _]
              tunnel: w226 -> [w234 _]
              frame True {
                n116 = invoke class="VI" method="FP.Open"(reference=w235, error in=w236, "State"=w234) -> (error out=w237:errorcluster)  [unwired: 2 in, 4 out]
              }
              frame False {
              }
            }
          }
          frame "Maximize", "Maximized" {
            w239 = T3."Maximized" ("State")
            n117 = property class="VI"(reference=w245, error in=w244) -> (reference out=w242:refnum<vi>, error out=w243:errorcluster, "FP.State"=w241:T3)
            n118 = Not Equal?(x=w241, y=w239) -> (x != y?=w240:bool)
            n119 = case shown="True" w240 {
              tunnel: [w250 w251] -> w246
              tunnel: w243 -> [w249 w251]
              tunnel: w242 -> [w248 _]
              tunnel: w239 -> [w247 _]
              frame True {
                n120 = invoke class="VI" method="FP.Open"(reference=w248, error in=w249, "State"=w247) -> (error out=w250:errorcluster)  [unwired: 2 in, 4 out]
              }
              frame False {
              }
            }
          }
        }
        n121 = call <vilib>:"Add State(s) to Queue__JKI_lib_State_Machine.vi"("State(s) in (\"\")"=w186) -> ("States Out"=w185:string)  [unwired: 14 in]
      }
      frame "---------- Macro ----------" {
        # "Do not put any code in this frame.\n(It is a separator no-op. You can make a copy of this frame to create a new Macro frame)"
        n122 = call <vilib>:"Add State(s) to Queue__JKI_lib_State_Machine.vi"("State(s) in (\"\")"=w255) -> ("States Out"=w254:string)  [unwired: 14 in]
      }
      frame "Macro: Initialize" {
        w256 = "Data: Initialize\nInitialize Core Data\nUI: Initialize\nUI: Front Panel State >> Open\nEvents: fclk\nEvents: On Controls\nEvents: Control"  # Data: Initialize Initialize Core Data UI: Initialize UI: Front Panel State >> Open Events: fclk Events: On Controls Events: Control
        # "Initialization Macro\n(This is called once, when the VI starts)"
        n123 = call <vilib>:"Add State(s) to Queue__JKI_lib_State_Machine.vi"("State(s) in Front (\"\")"=w256, "State(s) in (\"\")"=w260) -> ("States Out"=w259:string)  [unwired: 13 in]
      }
      frame "Macro: Exit" {
        # "Exit Macro\n(This is called once, when the VI exits)"
        n124 = Unbundle By Name(w267) -> ("Core.Close Panel on Exit?"=w266:bool)
        n125 = Select(t="UI: Front Panel State >> Close", s=w266, f="") -> (s? t:f=w263:string)
        n126 = call <vilib>:"Add State(s) to Queue__JKI_lib_State_Machine.vi"("State(s) in (\"\")"=w263, "State(s) at Back (\"\")"="Data: Cleanup\nExit") -> ("States Out"=w261:string)  [unwired: 13 in]
        n127 = call <vilib>:"Add State(s) to Queue__JKI_lib_State_Machine.vi"("State(s) in Front (\"\")"=w261, "State(s) in (\"\")"=w270) -> ("States Out"=w269:string)  [unwired: 13 in]
      }
      frame "---------- Events ----------" {
        # "Template Separator\n(You can make a copy of, or modify, this frame)"
        n128 = call <vilib>:"Add State(s) to Queue__JKI_lib_State_Machine.vi"("State(s) in (\"\")"=w274) -> ("States Out"=w273:string)  [unwired: 14 in]
      }
      frame "Events: Przetestuj" {
        # "Your code here.\n(You can make a copy of, or modify, this frame)"
        n129 = Unbundle By Name(w280) -> ("ClusterOUT.SygZad Podg Ref"=w279:refnum<vi>)
        n130 = disable-structure shown="Disabled" {
          frame Disabled {
            n131 = local read "Amplitude"() -> ()  [unwired: 1 out]
          }
          frame Enabled {
          }
        }
        n132 = property class="WFChart (strict)"(reference=w279, error in=w277, "History Data"=dynamicdata[] []) -> (reference out=w275:refnum<vi>, error out=w276:errorcluster)
        n133 = disable-structure shown="Disabled" {
          frame Disabled {
            n134 = local read "Offset SinZak"() -> ()  [unwired: 1 out]
            n135 = call "DistSignal.vi"() -> ()  [unwired: 15 in, 1 out]
          }
          frame Enabled {
          }
        }
        n136 = local read "Radio Buttons"() -> (w281:T2)
        n137 = Close Reference(reference=w275) -> ()  [unwired: 1 in, 1 out]
        n138 = case shown="\"Sygnał zakłócony\"" w281 {
          tunnel: [w291 w306 w314] -> w282
          tunnel: w276 -> [_ w307 _]
          frame "Sygnał przemienny", Default {
            n139 = local read "Offset"() -> (w287:dbl)
            n140 = local read "Frequency"() -> (w288:dbl)
            n141 = local read "Phase"() -> (w292:dbl)
            n142 = call "Simulate Signal"("Offset"=0.0, "Frequency"=w288, "Amplitude"=w287, "Phase"=w292) -> ("Sine"=w290:dynamicdata, "error out"=w291:errorcluster)  [unwired: 10 in]
            n143 = xnode "Set Dynamic Data Attributes"("Signals In"=w290) -> ("Signals Out"=w289:dynamicdata)  [unwired: 3 in, 1 out]
            n144 = local write "SygZad Podg"(w289) -> ()
          }
          frame "Sygnał zakłócony" {
            n145 = local read "Offset"() -> (w312:dbl)
            n146 = local read "Frequency"() -> (w311:dbl)
            n147 = local read "Amplitude"() -> (w310:dbl)
            n148 = local read "Phase"() -> (w309:dbl)
            n149 = call "Simulate Signal3"("Offset"=w312, "Frequency"=w311, "Amplitude"=w310, "Phase"=w309, "error in (no error)"=w307) -> ("Sine"=w308:dynamicdata, "error out"=w306:errorcluster)  [unwired: 9 in]
            n150 = local write "SygZad Podg"(w308) -> ()
          }
          frame "Sygnał stały" {
            n151 = local read "Offset"() -> (w317:dbl)
            n152 = call "Simulate Signal2"("Offset"=w317) -> ("DC"=w316:dynamicdata, "error out"=w315:errorcluster)  [unwired: 13 in]
            n153 = xnode "Set Dynamic Data Attributes"("Signals In"=w316, "error in"=w315) -> ("Signals Out"=→"SygZad Podg":dynamicdata, "error out"=w314:errorcluster)  [unwired: 2 in]
          }
        }
        n154 = call <vilib>:"Add State(s) to Queue__JKI_lib_State_Machine.vi"("State(s) in Front (\"\")"="Idle", "State(s) in (\"\")"=w285) -> ("States Out"=w284:string)  [unwired: 13 in]
      }
      frame "Events: Control" {
        # "Your code here.\n(You can make a copy of, or modify, this frame)"
        n155 = local read "Radio Buttons"() -> (w335:T2)
        n156 = case shown="\"Sygnał przemienny\", Default" w335 {
          tunnel: w334 -> [w339 w366 w389]
          tunnel: w333 -> [w350 w365 w385]
          tunnel: [w342 w355 w379] -> w332
          tunnel: ["Idle" "Idle" "Idle"] -> w331
          frame "Sygnał przemienny", Default {
            w338 = T5."Disabled and Grayed Out" ("Disabled")
            w351 = T5."Enabled" ("Disabled")
            n157 = Unbundle By Name(w339) -> ("ClusterOUT.Frequency Ref"=w354:refnum<vi>, "ClusterOUT.Amplitude Ref"=w353:refnum<vi>, "ClusterOUT.Phase Ref"=w352:refnum<vi>, "ClusterOUT.Offset sin zakłócającej Ref"=w344:refnum<vi>)
            n158 = property class="DigNum (strict)"(reference=w354, error in=w350, "DisabledEnum"=w351) -> (reference out=w348:refnum<vi>, error out=w349:errorcluster)
            n159 = property class="DigNum (strict)"(reference=w353, error in=w349, "DisabledEnum"=w338) -> (reference out=w346:refnum<vi>, error out=w347:errorcluster)
            n160 = property class="DigNum (strict)"(reference=w352, error in=w347, "DisabledEnum"=w351) -> (reference out=w345:refnum<vi>, error out=w343:errorcluster)
            n161 = property class="DigNum (strict)"(reference=w344, error in=w343, "DisabledEnum"=w338) -> (reference out=w341:refnum<vi>, error out=w342:errorcluster)
            n162 = Close Reference(reference=w346) -> ()  [unwired: 1 in, 1 out]
            n163 = Close Reference(reference=w348) -> ()  [unwired: 1 in, 1 out]
            n164 = Close Reference(reference=w341) -> ()  [unwired: 1 in, 1 out]
            n165 = Close Reference(reference=w345) -> ()  [unwired: 1 in, 1 out]
          }
          frame "Sygnał zakłócony" {
            w358 = T5."Enabled" ("Disabled")
            n166 = Unbundle By Name(w366) -> ("ClusterOUT.Frequency Ref"=w369:refnum<vi>, "ClusterOUT.Amplitude Ref"=w368:refnum<vi>, "ClusterOUT.Phase Ref"=w367:refnum<vi>, "ClusterOUT.Offset sin zakłócającej Ref"=w359:refnum<vi>)
            n167 = disable-structure shown="Enabled" {
              disable-tunnel: w359 -> [w372 w373]
              disable-tunnel: w358 -> [w371 _]
              disable-tunnel: [w370 w373] -> w357
              frame Disabled {
                n168 = property class="DigNum (strict)"(reference=w372, "DisabledEnum"=w371) -> (reference out=w370:refnum<vi>)  [unwired: 1 in, 1 out]
              }
              frame Enabled {
              }
            }
            n169 = property class="DigNum (strict)"(reference=w369, error in=w365, "DisabledEnum"=w358) -> (reference out=w363:refnum<vi>, error out=w364:errorcluster)
            n170 = property class="DigNum (strict)"(reference=w368, error in=w364, "DisabledEnum"=w358) -> (reference out=w361:refnum<vi>, error out=w362:errorcluster)
            n171 = property class="DigNum (strict)"(reference=w367, error in=w362, "DisabledEnum"=w358) -> (reference out=w360:refnum<vi>, error out=w355:errorcluster)
            n172 = Close Reference(reference=w361) -> ()  [unwired: 1 in, 1 out]
            n173 = Close Reference(reference=w363) -> ()  [unwired: 1 in, 1 out]
            n174 = Close Reference(reference=w357) -> ()  [unwired: 1 in, 1 out]
            n175 = Close Reference(reference=w360) -> ()  [unwired: 1 in, 1 out]
          }
          frame "Sygnał stały" {
            w381 = T5."Disabled and Grayed Out" ("Disabled")
            n176 = Unbundle By Name(w389) -> ("ClusterOUT.Frequency Ref"=w388:refnum<vi>, "ClusterOUT.Amplitude Ref"=w387:refnum<vi>, "ClusterOUT.Phase Ref"=w386:refnum<vi>, "ClusterOUT.Offset sin zakłócającej Ref"=w382:refnum<vi>)
            n177 = property class="DigNum (strict)"(reference=w388, error in=w385, "DisabledEnum"=w381) -> (reference out=w378:refnum<vi>, error out=w384:errorcluster)
            n178 = property class="DigNum (strict)"(reference=w387, error in=w384, "DisabledEnum"=w381) -> (reference out=w377:refnum<vi>, error out=w383:errorcluster)
            n179 = property class="DigNum (strict)"(reference=w386, error in=w383, "DisabledEnum"=w381) -> (reference out=w376:refnum<vi>, error out=w380:errorcluster)
            n180 = property class="DigNum (strict)"(reference=w382, error in=w380, "DisabledEnum"=w381) -> (reference out=w375:refnum<vi>, error out=w379:errorcluster)
            n181 = Close Reference(reference=w378) -> ()  [unwired: 1 in, 1 out]
            n182 = Close Reference(reference=w377) -> ()  [unwired: 1 in, 1 out]
            n183 = Close Reference(reference=w376) -> ()  [unwired: 1 in, 1 out]
            n184 = Close Reference(reference=w375) -> ()  [unwired: 1 in, 1 out]
          }
        }
        n185 = call <vilib>:"Add State(s) to Queue__JKI_lib_State_Machine.vi"("State(s) in Front (\"\")"=w331, "State(s) in (\"\")"=w337) -> ("States Out"=w336:string)  [unwired: 13 in]
      }
      frame "Events: knob" {
        # "Your code here.\n(You can make a copy of, or modify, this frame)"
        n186 = local read "fclkknob"() -> (w399:dbl)
        n187 = Unbundle By Name(w398) -> ("ClusterOUT.fclk-zad Ref"=w397:refnum<vi>)
        n188 = case shown="2" w399 {
          tunnel: w397 -> [w409 w417 w425 w433]
          tunnel: w396 -> [w407 w415 w423 w431]
          tunnel: [w402 w410 w418 w426] -> w393
          tunnel: ["Idle" "Idle" "Idle" "Idle"] -> w395
          tunnel: [w403 w413 w421 w429] -> w394
          frame 0, Default {
            w403 = 100.0 ("Value")
            n189 = property class="DigNum (strict)"(reference=w409, error in=w407, "Value"=w403, "DisabledEnum"=T5."Enabled" ("Disabled")) -> (reference out=w404:refnum<vi>, error out=w405:errorcluster)
            n190 = Close Reference(reference=w404, error in (no error)=w405) -> (error out=w402:errorcluster)
          }
          frame 1 {
            w413 = 100.0 ("Value")
            n191 = property class="DigNum (strict)"(reference=w417, error in=w415, "Value"=w413, "DisabledEnum"=T5."Disabled and Grayed Out" ("Disabled")) -> (reference out=w412:refnum<vi>, error out=w411:errorcluster)
            n192 = Close Reference(reference=w412, error in (no error)=w411) -> (error out=w410:errorcluster)
          }
          frame 2 {
            w421 = 500.0 ("Value")
            n193 = property class="DigNum (strict)"(reference=w425, error in=w423, "Value"=w421, "DisabledEnum"=T5."Disabled and Grayed Out" ("Disabled")) -> (reference out=w420:refnum<vi>, error out=w419:errorcluster)
            n194 = Close Reference(reference=w420, error in (no error)=w419) -> (error out=w418:errorcluster)
          }
          frame 3 {
            w429 = 35.0 ("Value")
            n195 = property class="DigNum (strict)"(reference=w433, error in=w431, "Value"=w429, "DisabledEnum"=T5."Enabled" ("Disabled")) -> (reference out=w428:refnum<vi>, error out=w427:errorcluster)
            n196 = Close Reference(reference=w428, error in (no error)=w427) -> (error out=w426:errorcluster)
          }
        }
        n197 = call "RateControl.vi"("error in (no error)"=w393, "Numeric"=w394) -> ("error out"=w390:errorcluster, "Numeric 3"=w391:u32, "Numeric 2"=w392:dbl)  [unwired: 7 in]
        n198 = local write "rate [Hz]"(w392) -> ()
        n199 = local write "Num of samp"(w391) -> ()
        n200 = call <vilib>:"Add State(s) to Queue__JKI_lib_State_Machine.vi"("State(s) in Front (\"\")"=w395, "State(s) in (\"\")"=w401) -> ("States Out"=w400:string)  [unwired: 13 in]
      }
      frame "Events: fclk" {
        # "Your code here.\n(You can make a copy of, or modify, this frame)"
        n201 = local read "fclk-zad"() -> (w437:dbl)
        n202 = call "RateControl.vi"("error in (no error)"=w438, "Numeric"=w437) -> ("error out"=w436:errorcluster, "Numeric 3"=w434:u32, "Numeric 2"=w435:dbl)  [unwired: 7 in]
        n203 = local write "rate [Hz]"(w435) -> ()
        n204 = local write "Num of samp"(w434) -> ()
        n205 = call <vilib>:"Add State(s) to Queue__JKI_lib_State_Machine.vi"("State(s) in (\"\")"=w441) -> ("States Out"=w440:string)  [unwired: 14 in]
      }
      frame "Events: check" {
        # "Your code here.\n(You can make a copy of, or modify, this frame)"
        n206 = local read "fclk-zad"() -> (w449:dbl)
        n207 = local read "Offset"() -> (w445:dbl)
        n208 = local read "Amplitude"() -> (w442:dbl)
        n209 = Greater?(x=w449, y=600.0) -> (0:w447:bool)
        n210 = case shown="True" w447 {
          selector: w447 -> [w461 w491]
          tunnel: [w462 w496] -> w446
          tunnel: w445 -> [w466 w495]
          tunnel: w444 -> [w464 w493]
          tunnel: [w456 w485] -> w443
          tunnel: w442 -> [w459 w489]
          frame True {
            w463 = "Za duza czestotliwosc!\n" ("Info")
            n211 = Greater?(x=w466, y=2.0) -> (0:w460:bool)
            n212 = Greater?(x=w459, y=0.2) -> (0:w454:bool)
            n213 = case shown="False" w460 {
              tunnel: w464 -> [w474 w478]
              tunnel: w463 -> [w477 w480]
              tunnel: [w474 w478] -> w457
              frame False {
                n214 = Concatenate Strings(w477, "" ("string")) -> (w476:string)
                n215 = local write "Info"(w476) -> ()
              }
              frame True {
                n216 = Concatenate Strings(w480, "Za duzy Offset!\n" ("Info")) -> (w481:string)
                n217 = local write "Info"(w481) -> ()
              }
            }
            n218 = Or(x=w461, y=w460) -> (x .or. y?=w455:bool)
            n219 = local write "Info"(w463) -> ()
            n220 = Or(x=w455, y=w454) -> (x .or. y?=w453:bool)
            n221 = case shown="True" w454 {
              tunnel: w457 -> [w467 w471]
              tunnel: [w467 w471] -> w456
              frame False {
              }
              frame True {
                n222 = local read "Info"() -> (w470:string)
                n223 = Concatenate Strings(w470, "Za duza amplituda!\n" ("string")) -> (w468:string)
                n224 = local write "Info"(w468) -> ()
              }
            }
            n225 = case shown="False" w453 {
              tunnel: ["Events: okres" "Idle"] -> w462
              frame False {
              }
              frame True {
              }
            }
          }
          frame False {
            w492 = "" ("Info")
            n226 = Greater?(x=w495, y=2.0) -> (0:w490:bool)
            n227 = case shown="True" w490 {
              tunnel: w493 -> [w506 w510]
              tunnel: w492 -> [w508 w512]
              tunnel: [w506 w510] -> w487
              frame True {
                n228 = Concatenate Strings(w508, "Za duzy Offset!\n" ("Info")) -> (w509:string)
                n229 = local write "Info"(w509) -> ()
              }
              frame False {
                n230 = Concatenate Strings(w512, "" ("Info")) -> (w513:string)
                n231 = local write "Info"(w513) -> ()
              }
            }
            n232 = local write "Info"(w492) -> ()
            n233 = call "Okres.vi"() -> ()  [unwired: 10 in, 2 out]
            n234 = Or(x=w491, y=w490) -> (x .or. y?=w482:bool)
            n235 = Greater?(x=w489, y=0.2) -> (0:w483:bool)
            n236 = Or(x=w482, y=w483) -> (x .or. y?=w484:bool)
            n237 = case shown="False" w483 {
              tunnel: w487 -> [w497 w501]
              tunnel: [w497 w501] -> w486
              frame False {
              }
              frame True {
                n238 = local read "Info"() -> (w500:string)
                n239 = Concatenate Strings(w500, "Za duza amplituda!\n" ("string")) -> (w498:string)
                n240 = local write "Info"(w498) -> ()
              }
            }
            n241 = case shown="True" w484 {
              tunnel: ["Events: okres" "Idle"] -> w496
              tunnel: w486 -> [w502 w504]
              tunnel: [w502 w504] -> w485
              frame False {
              }
              frame True {
              }
            }
          }
        }
        n242 = call <vilib>:"Add State(s) to Queue__JKI_lib_State_Machine.vi"("State(s) in Front (\"\")"=w446, "State(s) in (\"\")"=w452) -> ("States Out"=w451:string)  [unwired: 13 in]
      }
      frame "Events: okres" {
        # "Your code here.\n(You can make a copy of, or modify, this frame)"
        n243 = local read "fclk-zad"() -> (w528:dbl)
        n244 = local read "Uref"() -> (w548:dbl)
        n245 = local read "Offset"() -> (w547:dbl)
        n246 = call "Okres.vi"("error in (no error)"=w546, "Offset"=w547, "Uref"=w548, "fclk-zad"=w528) -> ("error out"=w524:errorcluster, "T1+T2"=w540:dbl)  [unwired: 6 in]
        "T1+T2" <- w540
        n247 = Number To Fractional String(number=w540) -> (F-format string=w536:string)  [unwired: 3 in]
        n248 = Multiply(x=w540, y=0.1) -> (x*y=w539:dbl)
        n249 = Add(x=w540, y=w539) -> (x+y=w533:dbl)
        n250 = control-ref of="INT IN"() -> (w545:refnum<vi>)
        n251 = control-ref of="IN HI / IN LO"() -> (w544:refnum<vi>)
        n252 = control-ref of="INT OUT"() -> (w543:refnum<vi>)
        n253 = control-ref of="COUNTER"() -> (w542:refnum<vi>)
        n254 = control-ref of="GATE"() -> (w541:refnum<vi>)
        n255 = call "RateControl.vi"("error in (no error)"=w524, "Numeric"=w528) -> ("error out"=w519:errorcluster, "Numeric 3"=w521:u32, "Numeric 2"=w527:dbl)  [unwired: 7 in]
        n256 = local write "BufPulse"(0.0 ("Numeric")) -> ()
        n257 = Concatenate Strings("Period of one cycle: " ("string"), w536, " second/s" ("string")) -> (w535:string)
        n258 = local write "rate [Hz]"(w527) -> ()
        n259 = local write "Num of samp"(w521) -> ()
        n260 = local write "Info"(w535) -> ()
        n261 = disable-structure shown="Disabled" {
          disable-tunnel: w533 -> [w570 _]
          disable-tunnel: [w568 _] -> _
          frame Disabled {
            n262 = Multiply(x=w570, y=5.0) -> (x*y=w568:dbl)
          }
          frame Enabled {
          }
        }
        n263 = disable-structure shown="Disabled" {
          disable-tunnel: w545 -> [w567 _]
          disable-tunnel: w544 -> [w566 _]
          disable-tunnel: w543 -> [w565 _]
          disable-tunnel: w542 -> [w564 _]
          disable-tunnel: w541 -> [w563 _]
          disable-tunnel: [w558 _] -> w526
          disable-tunnel: w524 -> [w557 _]
          frame Disabled {
            n264 = property class="WFChart (strict)" props=["XScale", "Maximum"](reference=w567, error in=w557) -> (reference out=w556:refnum<vi>, error out=w562:errorcluster)  [unwired: 1 in]
            n265 = property class="WFChart (strict)" props=["XScale", "Maximum"](reference=w566, error in=w562) -> (reference out=w555:refnum<vi>, error out=w561:errorcluster)  [unwired: 1 in]
            n266 = property class="WFChart (strict)" props=["XScale", "Maximum"](reference=w565, error in=w561) -> (reference out=w554:refnum<vi>, error out=w560:errorcluster)  [unwired: 1 in]
            n267 = property class="WFChart (strict)" props=["XScale", "Maximum"](reference=w564, error in=w560) -> (reference out=w553:refnum<vi>, error out=w559:errorcluster)  [unwired: 1 in]
            n268 = property class="WFChart (strict)" props=["XScale", "Maximum"](reference=w563, error in=w559) -> (reference out=w552:refnum<vi>, error out=w558:errorcluster)  [unwired: 1 in]
            n269 = Close Reference(reference=w556) -> ()  [unwired: 1 in, 1 out]
            n270 = Close Reference(reference=w552) -> ()  [unwired: 1 in, 1 out]
            n271 = Close Reference(reference=w555) -> ()  [unwired: 1 in, 1 out]
            n272 = Close Reference(reference=w554) -> ()  [unwired: 1 in, 1 out]
            n273 = Close Reference(reference=w553) -> ()  [unwired: 1 in, 1 out]
          }
          frame Enabled {
          }
        }
        n274 = control-ref of="IN HI/ IN LO"() -> (w532:refnum<vi>)
        n275 = control-ref of="INT OUT"() -> (w531:refnum<vi>)
        n276 = property class="WFGraph (strict)"(reference=w532, error in=w526, "XScale.Maximum"=1.0 ("X Scale.Range:Maximum"), "XScale.Minimum"=0.0 ("X Scale.Range:Minimum")) -> (reference out=w523:refnum<vi>, error out=w525:errorcluster)
        n277 = property class="WFGraph (strict)"(reference=w531, error in=w525, "XScale.Maximum"=1.0 ("X Scale.Range:Maximum"), "XScale.Minimum"=0.0 ("X Scale.Range:Minimum")) -> (reference out=w522:refnum<vi>, error out=w520:errorcluster)
        n278 = call <vilib>:"Add State(s) to Queue__JKI_lib_State_Machine.vi"("State(s) in Front (\"\")"="Events: Off Controls" ("State(s) in Front (\"\")"), "State(s) in (\"\")"=w551) -> ("States Out"=w550:string)  [unwired: 13 in]
        n279 = Close Reference(reference=w523) -> ()  [unwired: 1 in, 1 out]
        n280 = Merge Errors(w520, w519) -> (w518:errorcluster)
        n281 = Close Reference(reference=w522) -> ()  [unwired: 1 in, 1 out]
      }
      frame "Events: Charts Reset" {
        # "Initialize the User Interface, here.\n(this is called automatically, by the Macro: Init)"
        n282 = flat-sequence {
          tunnel: ["Events: Start"] -> w571
          frame #0 {
            w597 = dynamicdata[] [] ("History Data")
            n283 = control-ref of="IN HI / IN LO"() -> (w605:refnum<vi>)
            n284 = control-ref of="INT IN"() -> (w604:refnum<vi>)
            n285 = control-ref of="INT OUT"() -> (w603:refnum<vi>)
            n286 = control-ref of="GATE"() -> (w602:refnum<vi>)
            n287 = control-ref of="COUNTER"() -> (w601:refnum<vi>)
            n288 = control-ref of="INT OUT"() -> (w592:refnum<vi>)
            n289 = control-ref of="IN HI/ IN LO"() -> (w591:refnum<vi>)
            n290 = control-ref of="GATE"() -> (w590:refnum<vi>)
            n291 = control-ref of="INT IN"() -> (w589:refnum<vi>)
            n292 = control-ref of="COUNTER"() -> (w588:refnum<vi>)
            n293 = control-ref of="CE 2"() -> (w577:refnum<vi>)
            n294 = property class="WFGraph (strict)"(reference=w592, "Value"=0.0) -> (reference out=w587:refnum<vi>)  [unwired: 1 in, 1 out]
            n295 = property class="WFGraph (strict)"(reference=w591, "Value"=0.0) -> (reference out=w586:refnum<vi>)  [unwired: 1 in, 1 out]
            n296 = property class="WFGraph (strict)"(reference=w590, "Value"=0.0) -> (reference out=w585:refnum<vi>)  [unwired: 1 in, 1 out]
            n297 = property class="WFGraph (strict)"(reference=w589, "Value"=0.0) -> (reference out=w584:refnum<vi>)  [unwired: 1 in, 1 out]
            n298 = property class="WFGraph (strict)"(reference=w588, "Value"=dbl[] []) -> (reference out=w583:refnum<vi>)  [unwired: 1 in, 1 out]
            n299 = local write "COUNTER"(dbl[] array[295420 elements] ("COUNTER")) -> ()
            n300 = property class="WFChart (strict)"(reference=w577, "History Data"=dbl[] []) -> (reference out=w594:refnum<vi>)  [unwired: 1 in, 1 out]
            n301 = property class="WFChart (strict)"(reference=w605, "History Data"=w597) -> (reference out=w600:refnum<vi>)  [unwired: 1 in, 1 out]
            n302 = property class="WFChart (strict)"(reference=w604, "History Data"=w597) -> (reference out=w599:refnum<vi>)  [unwired: 1 in, 1 out]
            n303 = property class="WFChart (strict)"(reference=w603, "History Data"=w597) -> (reference out=w598:refnum<vi>)  [unwired: 1 in, 1 out]
            n304 = property class="WFChart (strict)"(reference=w602, "History Data"=w597) -> (reference out=w596:refnum<vi>)  [unwired: 1 in, 1 out]
            n305 = property class="WFChart (strict)"(reference=w601, "History Data"=w597) -> (reference out=w595:refnum<vi>)  [unwired: 1 in, 1 out]
            n306 = Close Reference(reference=w587) -> ()  [unwired: 1 in, 1 out]
            n307 = Close Reference(reference=w586) -> ()  [unwired: 1 in, 1 out]
            n308 = Close Reference(reference=w585) -> ()  [unwired: 1 in, 1 out]
            n309 = Close Reference(reference=w584) -> ()  [unwired: 1 in, 1 out]
            n310 = Close Reference(reference=w583) -> ()  [unwired: 1 in, 1 out]
            n311 = Close Reference(reference=w600) -> ()  [unwired: 1 in, 1 out]
            n312 = Close Reference(reference=w599) -> ()  [unwired: 1 in, 1 out]
            n313 = Close Reference(reference=w598) -> ()  [unwired: 1 in, 1 out]
            n314 = Close Reference(reference=w596) -> ()  [unwired: 1 in, 1 out]
            n315 = Close Reference(reference=w595) -> ()  [unwired: 1 in, 1 out]
            n316 = Close Reference(reference=w594) -> ()  [unwired: 1 in, 1 out]
          }
          frame #1 {
          }
        }
        n317 = call <vilib>:"Add State(s) to Queue__JKI_lib_State_Machine.vi"("State(s) in Front (\"\")"=w571, "State(s) in (\"\")"=w575) -> ("States Out"=w574:string)  [unwired: 13 in]
      }
      frame "Events: Off Controls" {
        w609 = T5."Disabled and Grayed Out" ("Disabled")
        w625 = T5."Disabled and Grayed Out" ("Disabled")
        # "Your code here.\n(You can make a copy of, or modify, this frame)"
        n318 = Unbundle By Name(w636) -> ("ClusterOUT.Radio Buttons Ref"=w635:refnum<vi>, "ClusterOUT.Test sygnału Ref"=w634:refnum<vi>, "ClusterOUT.Frequency Ref"=w633:refnum<vi>, "ClusterOUT.Amplitude Ref"=w632:refnum<vi>, "ClusterOUT.Phase Ref"=w631:refnum<vi>, "ClusterOUT.Offset Ref"=w630:refnum<vi>, "ClusterOUT.Offset sin zakłócającej Ref"=w629:refnum<vi>, "ClusterOUT.fclkknob Ref"=w628:refnum<vi>)  [unwired: 1 out]
        n319 = control-ref of="Uref"() -> (w626:refnum<vi>)
        n320 = control-ref of="Funk_pom"() -> (w627:refnum<vi>)
        n321 = property class="RadioBtnsControl (strict)"(reference=w635, "DisabledEnum"=w625) -> (reference out=w623:refnum<vi>)  [unwired: 1 in, 1 out]
        n322 = property class="Bool"(reference=w634, "DisabledEnum"=w625) -> (reference out=w622:refnum<vi>)  [unwired: 1 in, 1 out]
        n323 = property class="DigNum (strict)"(reference=w633, "DisabledEnum"=w625) -> (reference out=w621:refnum<vi>)  [unwired: 1 in, 1 out]
        n324 = property class="DigNum (strict)"(reference=w632, "DisabledEnum"=w625) -> (reference out=w620:refnum<vi>)  [unwired: 1 in, 1 out]
        n325 = property class="DigNum (strict)"(reference=w631, "DisabledEnum"=w625) -> (reference out=w619:refnum<vi>)  [unwired: 1 in, 1 out]
        n326 = property class="DigNum (strict)"(reference=w630, "DisabledEnum"=w625) -> (reference out=w618:refnum<vi>)  [unwired: 1 in, 1 out]
        n327 = property class="DigNum (strict)"(reference=w629, "DisabledEnum"=w625) -> (reference out=w617:refnum<vi>)  [unwired: 1 in, 1 out]
        n328 = property class="Knob (strict)"(reference=w628, "DisabledEnum"=w625) -> (reference out=w616:refnum<vi>)  [unwired: 1 in, 1 out]
        n329 = property class="RadioBtnsControl (strict)"(reference=w627, "DisabledEnum"=w625) -> (reference out=w615:refnum<vi>)  [unwired: 1 in, 1 out]
        n330 = property class="DigNum (strict)"(reference=w626, "DisabledEnum"=w625) -> (reference out=w614:refnum<vi>)  [unwired: 1 in, 1 out]
        n331 = Close Reference(reference=w623) -> ()  [unwired: 1 in, 1 out]
        n332 = Close Reference(reference=w622) -> ()  [unwired: 1 in, 1 out]
        n333 = Close Reference(reference=w621) -> ()  [unwired: 1 in, 1 out]
        n334 = Close Reference(reference=w620) -> ()  [unwired: 1 in, 1 out]
        n335 = Close Reference(reference=w619) -> ()  [unwired: 1 in, 1 out]
        n336 = Close Reference(reference=w618) -> ()  [unwired: 1 in, 1 out]
        n337 = Close Reference(reference=w617) -> ()  [unwired: 1 in, 1 out]
        n338 = Close Reference(reference=w616) -> ()  [unwired: 1 in, 1 out]
        n339 = Close Reference(reference=w615) -> ()  [unwired: 1 in, 1 out]
        n340 = Close Reference(reference=w614) -> ()  [unwired: 1 in, 1 out]
        n341 = control-ref of="Start Button"() -> (w610:refnum<vi>)
        n342 = control-ref of="Chart/Graph"() -> (w611:refnum<vi>)
        n343 = control-ref of="Exit Button"() -> (w613:refnum<vi>)
        n344 = property class="Bool (strict)"(reference=w611, "DisabledEnum"=w609) -> (reference out=w608:refnum<vi>)  [unwired: 1 in, 1 out]
        n345 = property class="Bool"(reference=w613, "DisabledEnum"=w609) -> (reference out=w612:refnum<vi>)  [unwired: 1 in, 1 out]
        n346 = property class="Bool"(reference=w610, "DisabledEnum"=w609) -> (reference out=w607:refnum<vi>)  [unwired: 1 in, 1 out]
        n347 = call <vilib>:"Add State(s) to Queue__JKI_lib_State_Machine.vi"("State(s) in Front (\"\")"="Events: Charts Reset" ("State(s) in Front (\"\")"), "State(s) in (\"\")"=w639) -> ("States Out"=w638:string)  [unwired: 13 in]
        n348 = Close Reference(reference=w612) -> ()  [unwired: 1 in, 1 out]
        n349 = Close Reference(reference=w607) -> ()  [unwired: 1 in, 1 out]
        n350 = Close Reference(reference=w608) -> ()  [unwired: 1 in, 1 out]
      }
      frame "Events: On Controls" {
        w640 = T5."Enabled" ("Disabled")
        w656 = T5."Enabled" ("Disabled")
        # "Your code here.\n(You can make a copy of, or modify, this frame)"
        n351 = Unbundle By Name(w667) -> ("ClusterOUT.Radio Buttons Ref"=w666:refnum<vi>, "ClusterOUT.Test sygnału Ref"=w665:refnum<vi>, "ClusterOUT.Frequency Ref"=w664:refnum<vi>, "ClusterOUT.Amplitude Ref"=w663:refnum<vi>, "ClusterOUT.Phase Ref"=w662:refnum<vi>, "ClusterOUT.Offset Ref"=w661:refnum<vi>, "ClusterOUT.Offset sin zakłócającej Ref"=w660:refnum<vi>, "ClusterOUT.fclkknob Ref"=w659:refnum<vi>)  [unwired: 1 out]
        n352 = control-ref of="Uref"() -> (w657:refnum<vi>)
        n353 = control-ref of="Funk_pom"() -> (w658:refnum<vi>)
        n354 = disable-structure shown="Enabled" {
          disable-tunnel: w660 -> [w672 w673]
          disable-tunnel: [w671 w673] -> w648
          frame Disabled {
            n355 = property class="DigNum (strict)" props=["DisabledEnum"](reference=w672) -> (reference out=w671:refnum<vi>)  [unwired: 2 in, 1 out]
          }
          frame Enabled {
          }
        }
        n356 = property class="RadioBtnsControl (strict)"(reference=w666, "DisabledEnum"=w656) -> (reference out=w654:refnum<vi>)  [unwired: 1 in, 1 out]
        n357 = property class="Bool"(reference=w665, "DisabledEnum"=w656) -> (reference out=w653:refnum<vi>)  [unwired: 1 in, 1 out]
        n358 = property class="DigNum (strict)"(reference=w664, "DisabledEnum"=w656) -> (reference out=w652:refnum<vi>)  [unwired: 1 in, 1 out]
        n359 = property class="DigNum (strict)"(reference=w663, "DisabledEnum"=w656) -> (reference out=w651:refnum<vi>)  [unwired: 1 in, 1 out]
        n360 = property class="DigNum (strict)"(reference=w662, "DisabledEnum"=w656) -> (reference out=w650:refnum<vi>)  [unwired: 1 in, 1 out]
        n361 = property class="DigNum (strict)"(reference=w661, "DisabledEnum"=w656) -> (reference out=w649:refnum<vi>)  [unwired: 1 in, 1 out]
        n362 = property class="Knob (strict)"(reference=w659, "DisabledEnum"=w656) -> (reference out=w647:refnum<vi>)  [unwired: 1 in, 1 out]
        n363 = property class="RadioBtnsControl (strict)"(reference=w658, "DisabledEnum"=w656) -> (reference out=w646:refnum<vi>)  [unwired: 1 in, 1 out]
        n364 = property class="DigNum (strict)"(reference=w657, "DisabledEnum"=w656) -> (reference out=w645:refnum<vi>)  [unwired: 1 in, 1 out]
        n365 = Close Reference(reference=w654) -> ()  [unwired: 1 in, 1 out]
        n366 = Close Reference(reference=w653) -> ()  [unwired: 1 in, 1 out]
        n367 = Close Reference(reference=w652) -> ()  [unwired: 1 in, 1 out]
        n368 = Close Reference(reference=w651) -> ()  [unwired: 1 in, 1 out]
        n369 = Close Reference(reference=w650) -> ()  [unwired: 1 in, 1 out]
        n370 = Close Reference(reference=w649) -> ()  [unwired: 1 in, 1 out]
        n371 = Close Reference(reference=w648) -> ()  [unwired: 1 in, 1 out]
        n372 = Close Reference(reference=w647) -> ()  [unwired: 1 in, 1 out]
        n373 = Close Reference(reference=w646) -> ()  [unwired: 1 in, 1 out]
        n374 = Close Reference(reference=w645) -> ()  [unwired: 1 in, 1 out]
        n375 = control-ref of="Exit Button"() -> (w644:refnum<vi>)
        n376 = control-ref of="Start Button"() -> (w641:refnum<vi>)
        n377 = control-ref of="Chart/Graph"() -> (w642:refnum<vi>)
        n378 = property class="Bool"(reference=w644, "DisabledEnum"=w640) -> (reference out=w643:refnum<vi>)  [unwired: 1 in, 1 out]
        n379 = property class="Bool (strict)"(reference=w642, "DisabledEnum"=w640) -> ()  [unwired: 1 in, 2 out]
        n380 = property class="Bool"(reference=w641, "DisabledEnum"=w640) -> ()  [unwired: 1 in, 2 out]
        n381 = call <vilib>:"Add State(s) to Queue__JKI_lib_State_Machine.vi"("State(s) in Front (\"\")"="Events: Control" ("State(s) in Front (\"\")"), "State(s) in (\"\")"=w670) -> ("States Out"=w669:string)  [unwired: 13 in]
        n382 = Close Reference(reference=w643) -> ()  [unwired: 1 in, 1 out]
      }
      frame "Events: Start" {
        # "CountEdges PIF2, ctr1"
        # "Your code here.\n(You can make a copy of, or modify, this frame)"
        n383 = local read "Offset"() -> (w695:dbl)
        n384 = local read "Frequency"() -> (w694:dbl)
        n385 = local read "Amplitude"() -> (w693:dbl)
        n386 = local read "Phase"() -> (w692:dbl)
        n387 = local read "Offset SinZak"() -> (w696:dbl)
        n388 = local read "Radio Buttons"() -> (w691:T2)
        n389 = local read "fclk-zad"() -> (w676:dbl)
        n390 = while {
          tunnel: w685 -> [w709]
          tunnel: [w705] -> w678
          tunnel: 1 ("number of samples") -> [w701]
          tunnel: "Funk_pom" -> [w702]
          stop <- w706 stop-if-true
          n391 = local read "Stop Button"() -> (w704:bool)
          n392 = global read "GlobalRes.vi" "Boolean"() -> (w710:bool)
          n393 = call "CountImpulse.vi"("error in"=w709, "stop (F)"=w704) -> ("error out"=w707:errorcluster, "stopped"=w708:bool, "Ilość impulsów"=w703:dbl)  [unwired: 7 in]
          n394 = case shown="\"F:1\"" w702 {
            tunnel: w710 -> [w717 w749]
            tunnel: w708 -> [w716 w747]
            tunnel: w707 -> [w715 w746]
            tunnel: [w714 w745] -> w706
            tunnel: [w713 w744] -> w705
            tunnel: w703 -> [w712 w748]
            tunnel: w701 -> [w711 w743]
            frame "F:1" {
              n395 = case shown="False" w717 {
                tunnel: w712 -> [w720 w731]
                tunnel: w716 -> [w722 w729]
                tunnel: w715 -> [w721 w728]
                tunnel: [w722 w725] -> w714
                tunnel: [w721 w724] -> w713
                tunnel: w711 -> [_ w723]
                frame False {
                  n396 = local read "BufPulse"() -> (w719:dbl)
                  n397 = Subtract(x=w720, y=w719) -> (x-y=→"CE 2":dbl)
                }
                frame True {
                  n398 = flat-sequence {
                    tunnel: w731 -> [w737]
                    tunnel: [w737] -> w730
                    tunnel: w729 -> [w736]
                    tunnel: w728 -> [w735]
                    tunnel: [w736] -> w727
                    tunnel: [w734] -> w726
                    tunnel: w723 -> [_]
                    tunnel: w730 -> [w742]
                    tunnel: w727 -> [w741]
                    tunnel: w726 -> [w740]
                    tunnel: [w741] -> w725
                    tunnel: [w740] -> w724
                    frame #0 {
                      n399 = local read "BufPulse"() -> (w738:dbl)
                      n400 = Subtract(x=w737, y=w738) -> (x-y=w732:dbl)
                      n401 = To Long Integer(number=w732) -> (32bit integer=w733:i32)
                      n402 = call "PlotPulses.vi"("error in (no error)"=w735, "Numeric"=w733) -> ("error out"=w734:errorcluster)  [unwired: 8 in, 1 out]
                      n403 = local write "Ilość impulsów"(w732) -> ()
                    }
                    frame #1 {
                      n404 = global write "GlobalRes.vi" "Boolean"(FALSE ("ResetCount")) -> ()
                      "BufPulse" <- w742
                    }
                  }
                }
              }
            }
            frame "F:2" {
              n405 = case shown="True" w749 {
                tunnel: w748 -> [_ w759]
                tunnel: w747 -> [w751 w758]
                tunnel: w746 -> [w750 w755]
                tunnel: [w751 w756] -> w745
                tunnel: [w750 w753] -> w744
                tunnel: w743 -> [_ w752]
                frame False {
                }
                frame True {
                  n406 = flat-sequence {
                    tunnel: w759 -> [w760]
                    tunnel: w758 -> [w765]
                    tunnel: [w765] -> w757
                    tunnel: w755 -> [w764]
                    tunnel: [w763] -> w754
                    tunnel: w752 -> [_]
                    tunnel: w757 -> [w767]
                    tunnel: [w767] -> w756
                    tunnel: w754 -> [w766]
                    tunnel: [w766] -> w753
                    frame #0 {
                      n407 = local write "CE 2"(w760) -> ()
                      n408 = local write "Ilość impulsów"(w760) -> ()
                      n409 = To Long Integer(number=w760) -> (32bit integer=w762:i32)
                      n410 = call "PlotPulses.vi"("error in (no error)"=w764, "Numeric"=w762) -> ("error out"=w763:errorcluster, "Waveform Graph 2"=w761:dbl[])  [unwired: 8 in]
                      n411 = local write "COUNTER"(w761) -> ()
                    }
                    frame #1 {
                      n412 = global write "GlobalRes.vi" "Boolean"(FALSE ("Boolean")) -> ()
                    }
                  }
                }
              }
            }
          }
        }
        n413 = local read "Ilosc_ai"() -> (w681:u8)
        n414 = call "TotalConvTime.vi"("fclk"=w676) -> ("TotalConvTime"=w675:dbl)  [unwired: 10 in]
        n415 = To Double Precision Float(number=w681) -> (double precision float=w680:dbl)
        n416 = call "Rate_Sample.vi"("Funk_pom"="Funk_pom", "Chart/Graph"="Chart/Graph", "Czas_cyklu"=w675, "ilosc_ai"=w680) -> ("Sample"=w682:i32, "Rate"=w683:dbl)  [unwired: 6 in]
        "Rate" <- w683
        "Number of samples" <- w682
        n417 = case shown="\"F:1\"" "Funk_pom" {
          selector: "Funk_pom" -> [w769 w782]
          tunnel: 1 ("number of samples") -> [w772 w785]
          tunnel: w685 -> [w771 w783]
          tunnel: [w770 w781] -> w684
          frame "F:1" {
            n418 = while {
              tunnel: w771 -> [w779]
              tunnel: w772 -> [w777]
              tunnel: [w776] -> w770
              tunnel: w769 -> [w774]
              stop <- w773 stop-if-true
              # "Gate PIF1, ctr0"
              n419 = local read "Stop Button"() -> (w775:bool)
              n420 = call "GateTime.vi"("error in"=w779, "Funk_pom"=w774, "stop (F)"=w775, "number of samples"=w777) -> ("error out"=w776:errorcluster, "stopped"=w773:bool, "Czas impulsu"=w778:dbl)  [unwired: 5 in]
              n421 = local write "Czas impulsu"(w778) -> ()
            }
          }
          frame "F:2" {
            # "Gate PIF1, ctr0"
            n422 = local read "Stop Button"() -> (w784:bool)
            n423 = call "GateTime.vi"("error in"=w783, "Funk_pom"=w782, "stop (F)"=w784, "number of samples"=w785) -> ("error out"=w781:errorcluster, "Czas impulsu"=w780:dbl)  [unwired: 5 in, 1 out]
            n424 = local write "Czas impulsu"(w780) -> ()
          }
        }
        n425 = case shown="\"F:1\", Default" "Funk_pom" {
          selector: "Funk_pom" -> [w789 w841]
          tunnel: [w791 w843] -> w689
          tunnel: w685 -> [w790 w842]
          tunnel: w683 -> [w788 w840]
          tunnel: w682 -> [w787 w839]
          tunnel: "Chart/Graph" -> [w786 w838]
          frame "F:1", Default {
            n426 = case shown="True" w786 {
              tunnel: w790 -> [w793 w816]
              tunnel: [w794 w817] -> w791
              tunnel: w788 -> [w797 w820]
              tunnel: w787 -> [w796 w819]
              tunnel: w789 -> [w795 w818]
              frame True {
                n427 = flat-sequence {
                  tunnel: w793 -> [w798]
                  tunnel: [w798] -> w792
                  frame #0 {
                    n428 = global write "GlobalRes.vi" "Boolean"(FALSE ("Boolean")) -> ()
                  }
                }
                n429 = while {
                  tunnel: w792 -> [w810]
                  tunnel: w797 -> [w812]
                  tunnel: w796 -> [w811]
                  tunnel: w795 -> [w805]
                  tunnel: [w807] -> w794
                  stop <- w806 stop-if-true
                  n430 = local read "Stop Button"() -> (w804:bool)
                  n431 = call "AcquireSingals.vi"("Funk_pom"=w805, "error in (no error)"=w810, "Stop Button"=w804, "Num of samp"=w811, "rate [Hz]"=w812) -> ("error out"=w808:errorcluster, "stopped"=w806:bool, "Waveform Chart"=w809:dynamicdata)  [unwired: 4 in]
                  n432 = Split Signals(w809) -> (→"IN HI / IN LO":dynamicdata, →"INT IN":dynamicdata, →"INT OUT":dynamicdata, →"GATE":dynamicdata)  [unwired: 5 in, 1 out]
                  n433 = flat-sequence {
                    tunnel: w808 -> [w813]
                    tunnel: [w813] -> w807
                    frame #0 {
                      n434 = global write "GlobalRes.vi" "Boolean"(TRUE ("Boolean")) -> ()
                    }
                  }
                }
              }
              frame False {
                n435 = flat-sequence {
                  tunnel: w816 -> [w821]
                  tunnel: [w821] -> w815
                  frame #0 {
                    n436 = global write "GlobalRes.vi" "Boolean"(FALSE ("Boolean")) -> ()
                  }
                }
                n437 = while {
                  tunnel: w820 -> [w832]
                  tunnel: w819 -> [w831]
                  tunnel: w818 -> [w830]
                  tunnel: [w828] -> w817
                  tunnel: w815 -> [w827]
                  stop <- w833 stop-if-true
                  n438 = local read "Stop Button"() -> (w835:bool)
                  n439 = call "AcquireSingals.vi"("Funk_pom"=w830, "error in (no error)"=w827, "Stop Button"=w835, "Num of samp"=w831, "rate [Hz]"=w832) -> ("error out"=w829:errorcluster, "stopped"=w833:bool, "Waveform Chart"=w834:dynamicdata)  [unwired: 4 in]
                  n440 = Split Signals(w834) -> (→"IN HI/ IN LO":dynamicdata, →"INT IN":dynamicdata, →"INT OUT":dynamicdata, →"GATE":dynamicdata)  [unwired: 5 in, 1 out]
                  n441 = flat-sequence {
                    tunnel: w829 -> [w836]
                    tunnel: [w836] -> w828
                    frame #0 {
                      n442 = global write "GlobalRes.vi" "Boolean"(TRUE ("Boolean")) -> ()
                    }
                  }
                }
              }
            }
          }
          frame "F:2" {
            n443 = case shown="False" w838 {
              tunnel: w842 -> [w851 w868]
              tunnel: [w848 w865] -> w843
              tunnel: w841 -> [w854 w869]
              tunnel: w840 -> [w853 w871]
              tunnel: w839 -> [w852 w870]
              frame True {
                n444 = flat-sequence {
                  tunnel: w851 -> [w860]
                  tunnel: [w860] -> w850
                  frame #0 {
                    n445 = global write "GlobalRes.vi" "Boolean"(FALSE ("Boolean")) -> ()
                  }
                }
                n446 = local read "Stop Button"() -> (w856:bool)
                n447 = call "AcquireSingals.vi"("Funk_pom"=w854, "error in (no error)"=w850, "Stop Button"=w856, "Num of samp"=w852, "rate [Hz]"=w853) -> ("error out"=w849:errorcluster, "Waveform Chart"=w855:dynamicdata)  [unwired: 4 in, 1 out]
                n448 = Split Signals(w855) -> (w847:dynamicdata, w846:dynamicdata, w845:dynamicdata, w844:dynamicdata)  [unwired: 5 in, 1 out]
                n449 = flat-sequence {
                  tunnel: w849 -> [w858]
                  tunnel: [w858] -> w848
                  frame #0 {
                    n450 = global write "GlobalRes.vi" "Boolean"(TRUE ("Boolean")) -> ()
                  }
                }
                n451 = local write "IN HI / IN LO"(w847) -> ()
                n452 = local write "GATE"(w844) -> ()
                n453 = local write "INT IN"(w846) -> ()
                n454 = local write "INT OUT"(w845) -> ()
              }
              frame False {
                n455 = flat-sequence {
                  tunnel: w868 -> [w876]
                  tunnel: [w876] -> w867
                  frame #0 {
                    n456 = global write "GlobalRes.vi" "Boolean"(FALSE ("Boolean")) -> ()
                  }
                }
                n457 = local read "Stop Button"() -> (w873:bool)
                n458 = call "AcquireSingals.vi"("Funk_pom"=w869, "error in (no error)"=w867, "Stop Button"=w873, "Num of samp"=w870, "rate [Hz]"=w871) -> ("error out"=w866:errorcluster, "Waveform Chart"=w872:dynamicdata)  [unwired: 4 in, 1 out]
                n459 = Split Signals(w872) -> (w864:dynamicdata, w863:dynamicdata, w862:dynamicdata, w861:dynamicdata)  [unwired: 5 in, 1 out]
                n460 = flat-sequence {
                  tunnel: w866 -> [w874]
                  tunnel: [w874] -> w865
                  frame #0 {
                    n461 = global write "GlobalRes.vi" "Boolean"(TRUE ("Boolean")) -> ()
                  }
                }
                n462 = local write "IN HI/ IN LO"(w864) -> ()
                n463 = local write "GATE"(w861) -> ()
                n464 = local write "INT IN"(w863) -> ()
                n465 = local write "INT OUT"(w862) -> ()
              }
            }
          }
        }
        n466 = while {
          tunnel: w696 -> [w887]
          tunnel: w695 -> [w886]
          tunnel: w694 -> [w885]
          tunnel: w693 -> [w884]
          tunnel: w692 -> [w883]
          tunnel: w691 -> [w882]
          tunnel: w685 -> [w881]
          tunnel: [w880] -> w690
          stop <- w879 stop-if-true
          n467 = call "GenerateSignal.vi"("Offset SinZak"=w887, "Offset"=w886, "Frequency"=w885, "Amplitude"=w884, "Phase"=w883, "Radio Buttons 2"=w882, "stop (F)"="Stop Button", "error in (no error)"=w881) -> ("stopped"=w879:bool, "error out"=w880:errorcluster)  [unwired: 18 in]
        }
        n468 = Merge Errors(w684, w690, w678, w689) -> (w687:errorcluster)
        n469 = flat-sequence {
          tunnel: ["Events: On Controls"] -> w697
          tunnel: w687 -> [w888]
          tunnel: [w888] -> w686
          frame #0 {
            n470 = local write "Stop Button"(FALSE ("Value")) -> ()
          }
        }
        n471 = call <vilib>:"Add State(s) to Queue__JKI_lib_State_Machine.vi"("State(s) in Front (\"\")"=w697, "State(s) in (\"\")"=w700) -> ("States Out"=w699:string)  [unwired: 13 in]
      }
    }
  }
